vi "Waveform 64-128 channels LP pt by pt.vi"(6 "order":i32=2, 8 "fl":dbl, 10 "fs":dbl, 11 "Array in":waveform(dbl)[](array[waveform])) -> (3 "Array out":waveform(dbl)[](array[waveform]))   [LabVIEW 2016]
uses:
  <vilib>/Analysis/3filter.llb/Filter Passband Type.ctl
  <vilib>/ptbypt/NI_PtbyPt.lvlib
  <vilib>/Analysis/NI_AALBase.lvlib
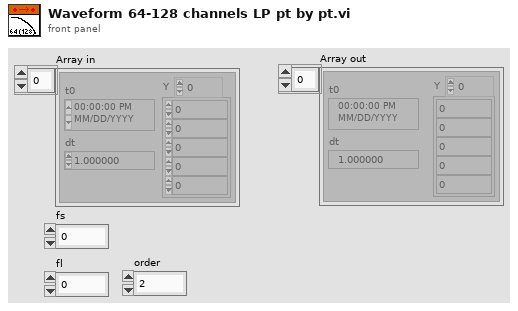
[diagram p1: front panel]
types:
  T1 = typedef "NI_AALBase.lvlib/Filter Passband Type.ctl" = enum32{"Lowpass", "Highpass", "Bandpass", "Bandstop"}
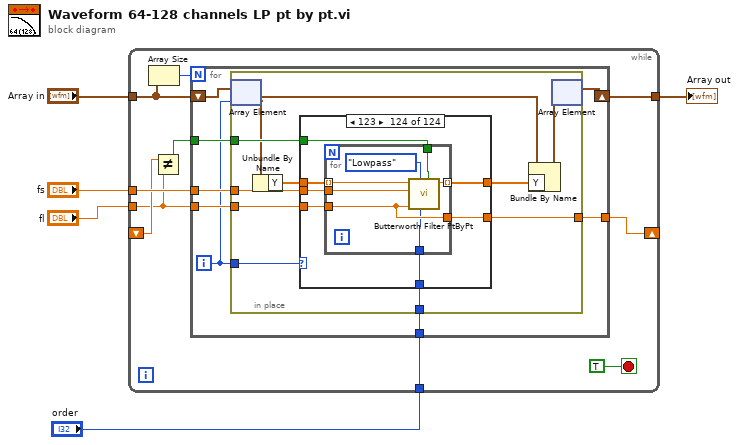
[diagram p0: block diagram]
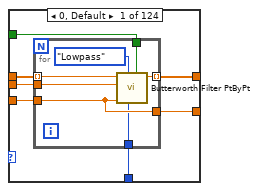
[diagram p2: hidden frame]
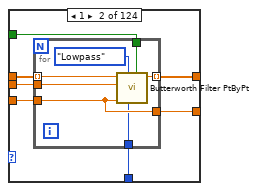
[diagram p3: hidden frame]
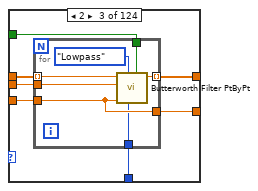
[diagram p4: hidden frame]
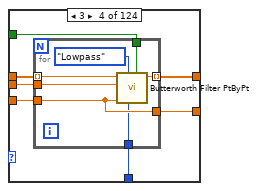
[diagram p5: hidden frame]
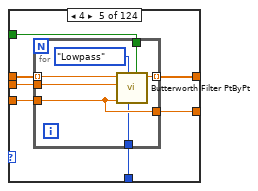
[diagram p6: hidden frame]
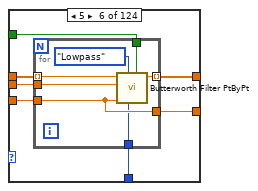
[diagram p7: hidden frame]
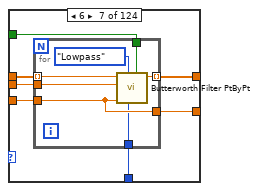
[diagram p8: hidden frame]
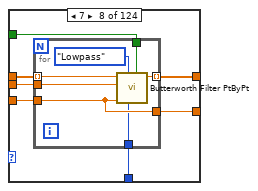
[diagram p9: hidden frame]
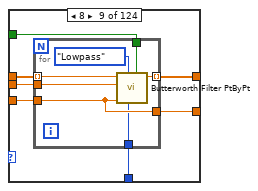
[diagram p10: hidden frame]
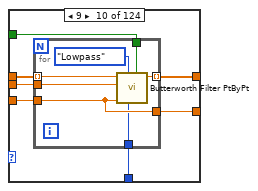
[diagram p11: hidden frame]
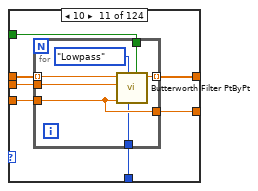
[diagram p12: hidden frame]
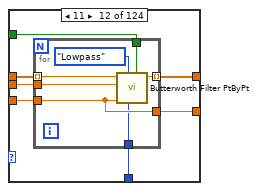
[diagram p13: hidden frame]
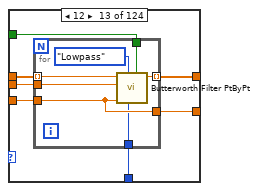
[diagram p14: hidden frame]
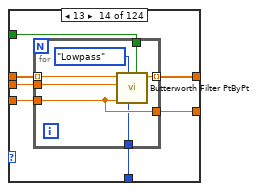
[diagram p15: hidden frame]
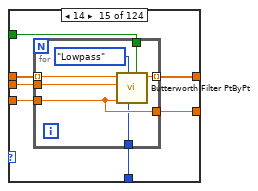
[diagram p16: hidden frame]
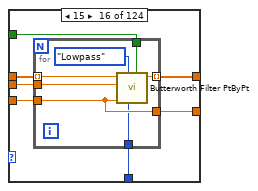
[diagram p17: hidden frame]
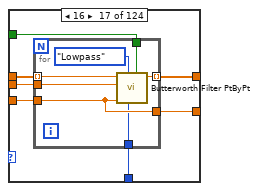
[diagram p18: hidden frame]
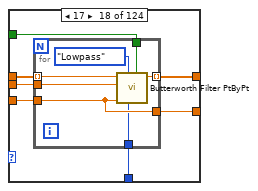
[diagram p19: hidden frame]
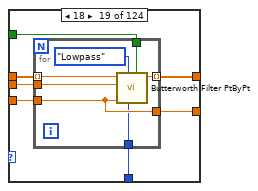
[diagram p20: hidden frame]
diagram:
  n1 = while {
    tunnel: "Array in" -> [w6]
    tunnel: [w15] -> w4
    tunnel: "fs" -> [w12]
    tunnel: "fl" -> [w9]
    shift-right: [w13] -> _
    shift-left: _ -> [w11]
    tunnel: "order" -> [w10]
    stop <- TRUE stop-if-true
    n2 = Array Size(array=w6) -> (size(s)=w7:i32)
    n3 = Not Equal?(x=w11, y=w9) -> (x != y?=w8:bool)
    n4 = for {
      N: w7 -> [_]
      tunnel: w12 -> [w23]
      tunnel: w9 -> [w22]
      tunnel: [w21] -> w13
      tunnel: w8 -> [w20]
      tunnel: w10 -> [w19]
      shift-right: [w16] -> w15
      shift-left: w6 -> [w18]
      i -> [w17]
      n5 = in-place {
        in-place-border: w23 -> [w33]
        in-place-border: w22 -> [w32]
        in-place-border: [w31] -> w21
        in-place-border: w20 -> [w30]
        in-place-border: w19 -> [w29]
        in-place-border: w17 -> [w26]
        n6 = in-place-array #1(w18, w17) -> (w25:waveform(dbl))
        n7 = Unbundle By Name(w25) -> ("Y"=w27:dbl[])
        n8 = case shown="123" w26 {
          tunnel: w33 -> [w40 w54 w68 w82 w96 w110 w124 w138 w152 w166 w180 w194 w208 w222 w236 w250 w264 w278 w292 w306 w320 w334 w348 w362 w376 w390 w404 w418 w432 w446 w460 w474 w488 w502 w516 w530 w544 w558 w572 w586 w600 w614 w628 w642 w656 w670 w684 w698 w712 w726 w740 w754 w768 w782 w796 w810 w824 w838 w852 w866 w880 w894 w908 w922 w936 w950 w964 w978 w992 w1006 w1020 w1034 w1048 w1062 w1076 w1090 w1104 w1118 w1132 w1146 w1160 w1174 w1188 w1202 w1216 w1230 w1244 w1258 w1272 w1286 w1300 w1314 w1328 w1342 w1356 w1370 w1384 w1398 w1412 w1426 w1440 w1454 w1468 w1482 w1496 w1510 w1524 w1538 w1552 w1566 w1580 w1594 w1608 w1622 w1636 w1650 w1664 w1678 w1692 w1706 w1720 w1734 w1748 w1762]
          tunnel: w32 -> [w39 w53 w67 w81 w95 w109 w123 w137 w151 w165 w179 w193 w207 w221 w235 w249 w263 w277 w291 w305 w319 w333 w347 w361 w375 w389 w403 w417 w431 w445 w459 w473 w487 w501 w515 w529 w543 w557 w571 w585 w599 w613 w627 w641 w655 w669 w683 w697 w711 w725 w739 w753 w767 w781 w795 w809 w823 w837 w851 w865 w879 w893 w907 w921 w935 w949 w963 w977 w991 w1005 w1019 w1033 w1047 w1061 w1075 w1089 w1103 w1117 w1131 w1145 w1159 w1173 w1187 w1201 w1215 w1229 w1243 w1257 w1271 w1285 w1299 w1313 w1327 w1341 w1355 w1369 w1383 w1397 w1411 w1425 w1439 w1453 w1467 w1481 w1495 w1509 w1523 w1537 w1551 w1565 w1579 w1593 w1607 w1621 w1635 w1649 w1663 w1677 w1691 w1705 w1719 w1733 w1747 w1761]
          tunnel: [w38 w52 w66 w80 w94 w108 w122 w136 w150 w164 w178 w192 w206 w220 w234 w248 w262 w276 w290 w304 w318 w332 w346 w360 w374 w388 w402 w416 w430 w444 w458 w472 w486 w500 w514 w528 w542 w556 w570 w584 w598 w612 w626 w640 w654 w668 w682 w696 w710 w724 w738 w752 w766 w780 w794 w808 w822 w836 w850 w864 w878 w892 w906 w920 w934 w948 w962 w976 w990 w1004 w1018 w1032 w1046 w1060 w1074 w1088 w1102 w1116 w1130 w1144 w1158 w1172 w1186 w1200 w1214 w1228 w1242 w1256 w1270 w1284 w1298 w1312 w1326 w1340 w1354 w1368 w1382 w1396 w1410 w1424 w1438 w1452 w1466 w1480 w1494 w1508 w1522 w1536 w1550 w1564 w1578 w1592 w1606 w1620 w1634 w1648 w1662 w1676 w1690 w1704 w1718 w1732 w1746 w1760] -> w31
          tunnel: w30 -> [w37 w51 w65 w79 w93 w107 w121 w135 w149 w163 w177 w191 w205 w219 w233 w247 w261 w275 w289 w303 w317 w331 w345 w359 w373 w387 w401 w415 w429 w443 w457 w471 w485 w499 w513 w527 w541 w555 w569 w583 w597 w611 w625 w639 w653 w667 w681 w695 w709 w723 w737 w751 w765 w779 w793 w807 w821 w835 w849 w863 w877 w891 w905 w919 w933 w947 w961 w975 w989 w1003 w1017 w1031 w1045 w1059 w1073 w1087 w1101 w1115 w1129 w1143 w1157 w1171 w1185 w1199 w1213 w1227 w1241 w1255 w1269 w1283 w1297 w1311 w1325 w1339 w1353 w1367 w1381 w1395 w1409 w1423 w1437 w1451 w1465 w1479 w1493 w1507 w1521 w1535 w1549 w1563 w1577 w1591 w1605 w1619 w1633 w1647 w1661 w1675 w1689 w1703 w1717 w1731 w1745 w1759]
          tunnel: w29 -> [w36 w50 w64 w78 w92 w106 w120 w134 w148 w162 w176 w190 w204 w218 w232 w246 w260 w274 w288 w302 w316 w330 w344 w358 w372 w386 w400 w414 w428 w442 w456 w470 w484 w498 w512 w526 w540 w554 w568 w582 w596 w610 w624 w638 w652 w666 w680 w694 w708 w722 w736 w750 w764 w778 w792 w806 w820 w834 w848 w862 w876 w890 w904 w918 w932 w946 w960 w974 w988 w1002 w1016 w1030 w1044 w1058 w1072 w1086 w1100 w1114 w1128 w1142 w1156 w1170 w1184 w1198 w1212 w1226 w1240 w1254 w1268 w1282 w1296 w1310 w1324 w1338 w1352 w1366 w1380 w1394 w1408 w1422 w1436 w1450 w1464 w1478 w1492 w1506 w1520 w1534 w1548 w1562 w1576 w1590 w1604 w1618 w1632 w1646 w1660 w1674 w1688 w1702 w1716 w1730 w1744 w1758]
          tunnel: [w35 w49 w63 w77 w91 w105 w119 w133 w147 w161 w175 w189 w203 w217 w231 w245 w259 w273 w287 w301 w315 w329 w343 w357 w371 w385 w399 w413 w427 w441 w455 w469 w483 w497 w511 w525 w539 w553 w567 w581 w595 w609 w623 w637 w651 w665 w679 w693 w707 w721 w735 w749 w763 w777 w791 w805 w819 w833 w847 w861 w875 w889 w903 w917 w931 w945 w959 w973 w987 w1001 w1015 w1029 w1043 w1057 w1071 w1085 w1099 w1113 w1127 w1141 w1155 w1169 w1183 w1197 w1211 w1225 w1239 w1253 w1267 w1281 w1295 w1309 w1323 w1337 w1351 w1365 w1379 w1393 w1407 w1421 w1435 w1449 w1463 w1477 w1491 w1505 w1519 w1533 w1547 w1561 w1575 w1589 w1603 w1617 w1631 w1645 w1659 w1673 w1687 w1701 w1715 w1729 w1743 w1757] -> w28
          tunnel: w27 -> [w34 w48 w62 w76 w90 w104 w118 w132 w146 w160 w174 w188 w202 w216 w230 w244 w258 w272 w286 w300 w314 w328 w342 w356 w370 w384 w398 w412 w426 w440 w454 w468 w482 w496 w510 w524 w538 w552 w566 w580 w594 w608 w622 w636 w650 w664 w678 w692 w706 w720 w734 w748 w762 w776 w790 w804 w818 w832 w846 w860 w874 w888 w902 w916 w930 w944 w958 w972 w986 w1000 w1014 w1028 w1042 w1056 w1070 w1084 w1098 w1112 w1126 w1140 w1154 w1168 w1182 w1196 w1210 w1224 w1238 w1252 w1266 w1280 w1294 w1308 w1322 w1336 w1350 w1364 w1378 w1392 w1406 w1420 w1434 w1448 w1462 w1476 w1490 w1504 w1518 w1532 w1546 w1560 w1574 w1588 w1602 w1616 w1630 w1644 w1658 w1672 w1686 w1700 w1714 w1728 w1742 w1756]
          frame 0, Default {
            n9 = for {
              tunnel: w34 -> [w47] mode=indexing
              tunnel: w39 -> [w44]
              tunnel: w40 -> [w46]
              tunnel: [w45] -> w35 mode=indexing
              tunnel: [w44] -> w38
              tunnel: w37 -> [w42]
              tunnel: w36 -> [w41]
              n10 = call <vilib>:"Butterworth Filter PtByPt.vi"("initialize"=w42, "order"=w41, "filter type"=Filter_Passband_Type."Lowpass", "low cutoff freq: fl"=w44, "sampling freq: fs"=w46, "x"=w47) -> ("Filtered x"=w45:dbl)  [unwired: 3 in, 1 out]
            }
          }
          frame 1 {
            n11 = for {
              tunnel: w48 -> [w61] mode=indexing
              tunnel: w53 -> [w58]
              tunnel: w54 -> [w60]
              tunnel: [w59] -> w49 mode=indexing
              tunnel: [w58] -> w52
              tunnel: w51 -> [w56]
              tunnel: w50 -> [w55]
              n12 = call <vilib>:"Butterworth Filter PtByPt.vi"("initialize"=w56, "order"=w55, "filter type"=Filter_Passband_Type."Lowpass", "low cutoff freq: fl"=w58, "sampling freq: fs"=w60, "x"=w61) -> ("Filtered x"=w59:dbl)  [unwired: 3 in, 1 out]
            }
          }
          frame 2 {
            n13 = for {
              tunnel: w62 -> [w75] mode=indexing
              tunnel: w67 -> [w72]
              tunnel: w68 -> [w74]
              tunnel: [w73] -> w63 mode=indexing
              tunnel: [w72] -> w66
              tunnel: w65 -> [w70]
              tunnel: w64 -> [w69]
              n14 = call <vilib>:"Butterworth Filter PtByPt.vi"("initialize"=w70, "order"=w69, "filter type"=Filter_Passband_Type."Lowpass", "low cutoff freq: fl"=w72, "sampling freq: fs"=w74, "x"=w75) -> ("Filtered x"=w73:dbl)  [unwired: 3 in, 1 out]
            }
          }
          frame 3 {
            n15 = for {
              tunnel: w76 -> [w89] mode=indexing
              tunnel: w81 -> [w86]
              tunnel: w82 -> [w88]
              tunnel: [w87] -> w77 mode=indexing
              tunnel: [w86] -> w80
              tunnel: w79 -> [w84]
              tunnel: w78 -> [w83]
              n16 = call <vilib>:"Butterworth Filter PtByPt.vi"("initialize"=w84, "order"=w83, "filter type"=Filter_Passband_Type."Lowpass", "low cutoff freq: fl"=w86, "sampling freq: fs"=w88, "x"=w89) -> ("Filtered x"=w87:dbl)  [unwired: 3 in, 1 out]
            }
          }
          frame 4 {
            n17 = for {
              tunnel: w90 -> [w103] mode=indexing
              tunnel: w95 -> [w100]
              tunnel: w96 -> [w102]
              tunnel: [w101] -> w91 mode=indexing
              tunnel: [w100] -> w94
              tunnel: w93 -> [w98]
              tunnel: w92 -> [w97]
              n18 = call <vilib>:"Butterworth Filter PtByPt.vi"("initialize"=w98, "order"=w97, "filter type"=Filter_Passband_Type."Lowpass", "low cutoff freq: fl"=w100, "sampling freq: fs"=w102, "x"=w103) -> ("Filtered x"=w101:dbl)  [unwired: 3 in, 1 out]
            }
          }
          frame 5 {
            n19 = for {
              tunnel: w104 -> [w117] mode=indexing
              tunnel: w109 -> [w114]
              tunnel: w110 -> [w116]
              tunnel: [w115] -> w105 mode=indexing
              tunnel: [w114] -> w108
              tunnel: w107 -> [w112]
              tunnel: w106 -> [w111]
              n20 = call <vilib>:"Butterworth Filter PtByPt.vi"("initialize"=w112, "order"=w111, "filter type"=Filter_Passband_Type."Lowpass", "low cutoff freq: fl"=w114, "sampling freq: fs"=w116, "x"=w117) -> ("Filtered x"=w115:dbl)  [unwired: 3 in, 1 out]
            }
          }
          frame 6 {
            n21 = for {
              tunnel: w118 -> [w131] mode=indexing
              tunnel: w123 -> [w128]
              tunnel: w124 -> [w130]
              tunnel: [w129] -> w119 mode=indexing
              tunnel: [w128] -> w122
              tunnel: w121 -> [w126]
              tunnel: w120 -> [w125]
              n22 = call <vilib>:"Butterworth Filter PtByPt.vi"("initialize"=w126, "order"=w125, "filter type"=Filter_Passband_Type."Lowpass", "low cutoff freq: fl"=w128, "sampling freq: fs"=w130, "x"=w131) -> ("Filtered x"=w129:dbl)  [unwired: 3 in, 1 out]
            }
          }
          frame 7 {
            n23 = for {
              tunnel: w132 -> [w145] mode=indexing
              tunnel: w137 -> [w142]
              tunnel: w138 -> [w144]
              tunnel: [w143] -> w133 mode=indexing
              tunnel: [w142] -> w136
              tunnel: w135 -> [w140]
              tunnel: w134 -> [w139]
              n24 = call <vilib>:"Butterworth Filter PtByPt.vi"("initialize"=w140, "order"=w139, "filter type"=Filter_Passband_Type."Lowpass", "low cutoff freq: fl"=w142, "sampling freq: fs"=w144, "x"=w145) -> ("Filtered x"=w143:dbl)  [unwired: 3 in, 1 out]
            }
          }
          frame 8 {
            n25 = for {
              tunnel: w146 -> [w159] mode=indexing
              tunnel: w151 -> [w156]
              tunnel: w152 -> [w158]
              tunnel: [w157] -> w147 mode=indexing
              tunnel: [w156] -> w150
              tunnel: w149 -> [w154]
              tunnel: w148 -> [w153]
              n26 = call <vilib>:"Butterworth Filter PtByPt.vi"("initialize"=w154, "order"=w153, "filter type"=Filter_Passband_Type."Lowpass", "low cutoff freq: fl"=w156, "sampling freq: fs"=w158, "x"=w159) -> ("Filtered x"=w157:dbl)  [unwired: 3 in, 1 out]
            }
          }
          frame 9 {
            n27 = for {
              tunnel: w160 -> [w173] mode=indexing
              tunnel: w165 -> [w170]
              tunnel: w166 -> [w172]
              tunnel: [w171] -> w161 mode=indexing
              tunnel: [w170] -> w164
              tunnel: w163 -> [w168]
              tunnel: w162 -> [w167]
              n28 = call <vilib>:"Butterworth Filter PtByPt.vi"("initialize"=w168, "order"=w167, "filter type"=Filter_Passband_Type."Lowpass", "low cutoff freq: fl"=w170, "sampling freq: fs"=w172, "x"=w173) -> ("Filtered x"=w171:dbl)  [unwired: 3 in, 1 out]
            }
          }
          frame 10 {
            n29 = for {
              tunnel: w174 -> [w187] mode=indexing
              tunnel: w179 -> [w184]
              tunnel: w180 -> [w186]
              tunnel: [w185] -> w175 mode=indexing
              tunnel: [w184] -> w178
              tunnel: w177 -> [w182]
              tunnel: w176 -> [w181]
              n30 = call <vilib>:"Butterworth Filter PtByPt.vi"("initialize"=w182, "order"=w181, "filter type"=Filter_Passband_Type."Lowpass", "low cutoff freq: fl"=w184, "sampling freq: fs"=w186, "x"=w187) -> ("Filtered x"=w185:dbl)  [unwired: 3 in, 1 out]
            }
          }
          frame 11 {
            n31 = for {
              tunnel: w188 -> [w201] mode=indexing
              tunnel: w193 -> [w198]
              tunnel: w194 -> [w200]
              tunnel: [w199] -> w189 mode=indexing
              tunnel: [w198] -> w192
              tunnel: w191 -> [w196]
              tunnel: w190 -> [w195]
              n32 = call <vilib>:"Butterworth Filter PtByPt.vi"("initialize"=w196, "order"=w195, "filter type"=Filter_Passband_Type."Lowpass", "low cutoff freq: fl"=w198, "sampling freq: fs"=w200, "x"=w201) -> ("Filtered x"=w199:dbl)  [unwired: 3 in, 1 out]
            }
          }
          frame 12 {
            n33 = for {
              tunnel: w202 -> [w215] mode=indexing
              tunnel: w207 -> [w212]
              tunnel: w208 -> [w214]
              tunnel: [w213] -> w203 mode=indexing
              tunnel: [w212] -> w206
              tunnel: w205 -> [w210]
              tunnel: w204 -> [w209]
              n34 = call <vilib>:"Butterworth Filter PtByPt.vi"("initialize"=w210, "order"=w209, "filter type"=Filter_Passband_Type."Lowpass", "low cutoff freq: fl"=w212, "sampling freq: fs"=w214, "x"=w215) -> ("Filtered x"=w213:dbl)  [unwired: 3 in, 1 out]
            }
          }
          frame 13 {
            n35 = for {
              tunnel: w216 -> [w229] mode=indexing
              tunnel: w221 -> [w226]
              tunnel: w222 -> [w228]
              tunnel: [w227] -> w217 mode=indexing
              tunnel: [w226] -> w220
              tunnel: w219 -> [w224]
              tunnel: w218 -> [w223]
              n36 = call <vilib>:"Butterworth Filter PtByPt.vi"("initialize"=w224, "order"=w223, "filter type"=Filter_Passband_Type."Lowpass", "low cutoff freq: fl"=w226, "sampling freq: fs"=w228, "x"=w229) -> ("Filtered x"=w227:dbl)  [unwired: 3 in, 1 out]
            }
          }
          frame 14 {
            n37 = for {
              tunnel: w230 -> [w243] mode=indexing
              tunnel: w235 -> [w240]
              tunnel: w236 -> [w242]
              tunnel: [w241] -> w231 mode=indexing
              tunnel: [w240] -> w234
              tunnel: w233 -> [w238]
              tunnel: w232 -> [w237]
              n38 = call <vilib>:"Butterworth Filter PtByPt.vi"("initialize"=w238, "order"=w237, "filter type"=Filter_Passband_Type."Lowpass", "low cutoff freq: fl"=w240, "sampling freq: fs"=w242, "x"=w243) -> ("Filtered x"=w241:dbl)  [unwired: 3 in, 1 out]
            }
          }
          frame 15 {
            n39 = for {
              tunnel: w244 -> [w257] mode=indexing
              tunnel: w249 -> [w254]
              tunnel: w250 -> [w256]
              tunnel: [w255] -> w245 mode=indexing
              tunnel: [w254] -> w248
              tunnel: w247 -> [w252]
              tunnel: w246 -> [w251]
              n40 = call <vilib>:"Butterworth Filter PtByPt.vi"("initialize"=w252, "order"=w251, "filter type"=Filter_Passband_Type."Lowpass", "low cutoff freq: fl"=w254, "sampling freq: fs"=w256, "x"=w257) -> ("Filtered x"=w255:dbl)  [unwired: 3 in, 1 out]
            }
          }
          frame 16 {
            n41 = for {
              tunnel: w258 -> [w271] mode=indexing
              tunnel: w263 -> [w268]
              tunnel: w264 -> [w270]
              tunnel: [w269] -> w259 mode=indexing
              tunnel: [w268] -> w262
              tunnel: w261 -> [w266]
              tunnel: w260 -> [w265]
              n42 = call <vilib>:"Butterworth Filter PtByPt.vi"("initialize"=w266, "order"=w265, "filter type"=Filter_Passband_Type."Lowpass", "low cutoff freq: fl"=w268, "sampling freq: fs"=w270, "x"=w271) -> ("Filtered x"=w269:dbl)  [unwired: 3 in, 1 out]
            }
          }
          frame 17 {
            n43 = for {
              tunnel: w272 -> [w285] mode=indexing
              tunnel: w277 -> [w282]
              tunnel: w278 -> [w284]
              tunnel: [w283] -> w273 mode=indexing
              tunnel: [w282] -> w276
              tunnel: w275 -> [w280]
              tunnel: w274 -> [w279]
              n44 = call <vilib>:"Butterworth Filter PtByPt.vi"("initialize"=w280, "order"=w279, "filter type"=Filter_Passband_Type."Lowpass", "low cutoff freq: fl"=w282, "sampling freq: fs"=w284, "x"=w285) -> ("Filtered x"=w283:dbl)  [unwired: 3 in, 1 out]
            }
          }
          frame 18 {
            n45 = for {
              tunnel: w286 -> [w299] mode=indexing
              tunnel: w291 -> [w296]
              tunnel: w292 -> [w298]
              tunnel: [w297] -> w287 mode=indexing
              tunnel: [w296] -> w290
              tunnel: w289 -> [w294]
              tunnel: w288 -> [w293]
              n46 = call <vilib>:"Butterworth Filter PtByPt.vi"("initialize"=w294, "order"=w293, "filter type"=Filter_Passband_Type."Lowpass", "low cutoff freq: fl"=w296, "sampling freq: fs"=w298, "x"=w299) -> ("Filtered x"=w297:dbl)  [unwired: 3 in, 1 out]
            }
          }
          frame 19 {
            n47 = for {
              tunnel: w300 -> [w313] mode=indexing
              tunnel: w305 -> [w310]
              tunnel: w306 -> [w312]
              tunnel: [w311] -> w301 mode=indexing
              tunnel: [w310] -> w304
              tunnel: w303 -> [w308]
              tunnel: w302 -> [w307]
              n48 = call <vilib>:"Butterworth Filter PtByPt.vi"("initialize"=w308, "order"=w307, "filter type"=Filter_Passband_Type."Lowpass", "low cutoff freq: fl"=w310, "sampling freq: fs"=w312, "x"=w313) -> ("Filtered x"=w311:dbl)  [unwired: 3 in, 1 out]
            }
          }
          frame 20 {
            n49 = for {
              tunnel: w314 -> [w327] mode=indexing
              tunnel: w319 -> [w324]
              tunnel: w320 -> [w326]
              tunnel: [w325] -> w315 mode=indexing
              tunnel: [w324] -> w318
              tunnel: w317 -> [w322]
              tunnel: w316 -> [w321]
              n50 = call <vilib>:"Butterworth Filter PtByPt.vi"("initialize"=w322, "order"=w321, "filter type"=Filter_Passband_Type."Lowpass", "low cutoff freq: fl"=w324, "sampling freq: fs"=w326, "x"=w327) -> ("Filtered x"=w325:dbl)  [unwired: 3 in, 1 out]
            }
          }
          frame 21 {
            n51 = for {
              tunnel: w328 -> [w341] mode=indexing
              tunnel: w333 -> [w338]
              tunnel: w334 -> [w340]
              tunnel: [w339] -> w329 mode=indexing
              tunnel: [w338] -> w332
              tunnel: w331 -> [w336]
              tunnel: w330 -> [w335]
              n52 = call <vilib>:"Butterworth Filter PtByPt.vi"("initialize"=w336, "order"=w335, "filter type"=Filter_Passband_Type."Lowpass", "low cutoff freq: fl"=w338, "sampling freq: fs"=w340, "x"=w341) -> ("Filtered x"=w339:dbl)  [unwired: 3 in, 1 out]
            }
          }
          frame 22 {
            n53 = for {
              tunnel: w342 -> [w355] mode=indexing
              tunnel: w347 -> [w352]
              tunnel: w348 -> [w354]
              tunnel: [w353] -> w343 mode=indexing
              tunnel: [w352] -> w346
              tunnel: w345 -> [w350]
              tunnel: w344 -> [w349]
              n54 = call <vilib>:"Butterworth Filter PtByPt.vi"("initialize"=w350, "order"=w349, "filter type"=Filter_Passband_Type."Lowpass", "low cutoff freq: fl"=w352, "sampling freq: fs"=w354, "x"=w355) -> ("Filtered x"=w353:dbl)  [unwired: 3 in, 1 out]
            }
          }
          frame 23 {
            n55 = for {
              tunnel: w356 -> [w369] mode=indexing
              tunnel: w361 -> [w366]
              tunnel: w362 -> [w368]
              tunnel: [w367] -> w357 mode=indexing
              tunnel: [w366] -> w360
              tunnel: w359 -> [w364]
              tunnel: w358 -> [w363]
              n56 = call <vilib>:"Butterworth Filter PtByPt.vi"("initialize"=w364, "order"=w363, "filter type"=Filter_Passband_Type."Lowpass", "low cutoff freq: fl"=w366, "sampling freq: fs"=w368, "x"=w369) -> ("Filtered x"=w367:dbl)  [unwired: 3 in, 1 out]
            }
          }
          frame 24 {
            n57 = for {
              tunnel: w370 -> [w383] mode=indexing
              tunnel: w375 -> [w380]
              tunnel: w376 -> [w382]
              tunnel: [w381] -> w371 mode=indexing
              tunnel: [w380] -> w374
              tunnel: w373 -> [w378]
              tunnel: w372 -> [w377]
              n58 = call <vilib>:"Butterworth Filter PtByPt.vi"("initialize"=w378, "order"=w377, "filter type"=Filter_Passband_Type."Lowpass", "low cutoff freq: fl"=w380, "sampling freq: fs"=w382, "x"=w383) -> ("Filtered x"=w381:dbl)  [unwired: 3 in, 1 out]
            }
          }
          frame 25 {
            n59 = for {
              tunnel: w384 -> [w397] mode=indexing
              tunnel: w389 -> [w394]
              tunnel: w390 -> [w396]
              tunnel: [w395] -> w385 mode=indexing
              tunnel: [w394] -> w388
              tunnel: w387 -> [w392]
              tunnel: w386 -> [w391]
              n60 = call <vilib>:"Butterworth Filter PtByPt.vi"("initialize"=w392, "order"=w391, "filter type"=Filter_Passband_Type."Lowpass", "low cutoff freq: fl"=w394, "sampling freq: fs"=w396, "x"=w397) -> ("Filtered x"=w395:dbl)  [unwired: 3 in, 1 out]
            }
          }
          frame 26 {
            n61 = for {
              tunnel: w398 -> [w411] mode=indexing
              tunnel: w403 -> [w408]
              tunnel: w404 -> [w410]
              tunnel: [w409] -> w399 mode=indexing
              tunnel: [w408] -> w402
              tunnel: w401 -> [w406]
              tunnel: w400 -> [w405]
              n62 = call <vilib>:"Butterworth Filter PtByPt.vi"("initialize"=w406, "order"=w405, "filter type"=Filter_Passband_Type."Lowpass", "low cutoff freq: fl"=w408, "sampling freq: fs"=w410, "x"=w411) -> ("Filtered x"=w409:dbl)  [unwired: 3 in, 1 out]
            }
          }
          frame 27 {
            n63 = for {
              tunnel: w412 -> [w425] mode=indexing
              tunnel: w417 -> [w422]
              tunnel: w418 -> [w424]
              tunnel: [w423] -> w413 mode=indexing
              tunnel: [w422] -> w416
              tunnel: w415 -> [w420]
              tunnel: w414 -> [w419]
              n64 = call <vilib>:"Butterworth Filter PtByPt.vi"("initialize"=w420, "order"=w419, "filter type"=Filter_Passband_Type."Lowpass", "low cutoff freq: fl"=w422, "sampling freq: fs"=w424, "x"=w425) -> ("Filtered x"=w423:dbl)  [unwired: 3 in, 1 out]
            }
          }
          frame 28 {
            n65 = for {
              tunnel: w426 -> [w439] mode=indexing
              tunnel: w431 -> [w436]
              tunnel: w432 -> [w438]
              tunnel: [w437] -> w427 mode=indexing
              tunnel: [w436] -> w430
              tunnel: w429 -> [w434]
              tunnel: w428 -> [w433]
              n66 = call <vilib>:"Butterworth Filter PtByPt.vi"("initialize"=w434, "order"=w433, "filter type"=Filter_Passband_Type."Lowpass", "low cutoff freq: fl"=w436, "sampling freq: fs"=w438, "x"=w439) -> ("Filtered x"=w437:dbl)  [unwired: 3 in, 1 out]
            }
          }
          frame 29 {
            n67 = for {
              tunnel: w440 -> [w453] mode=indexing
              tunnel: w445 -> [w450]
              tunnel: w446 -> [w452]
              tunnel: [w451] -> w441 mode=indexing
              tunnel: [w450] -> w444
              tunnel: w443 -> [w448]
              tunnel: w442 -> [w447]
              n68 = call <vilib>:"Butterworth Filter PtByPt.vi"("initialize"=w448, "order"=w447, "filter type"=Filter_Passband_Type."Lowpass", "low cutoff freq: fl"=w450, "sampling freq: fs"=w452, "x"=w453) -> ("Filtered x"=w451:dbl)  [unwired: 3 in, 1 out]
            }
          }
          frame 30 {
            n69 = for {
              tunnel: w454 -> [w467] mode=indexing
              tunnel: w459 -> [w464]
              tunnel: w460 -> [w466]
              tunnel: [w465] -> w455 mode=indexing
              tunnel: [w464] -> w458
              tunnel: w457 -> [w462]
              tunnel: w456 -> [w461]
              n70 = call <vilib>:"Butterworth Filter PtByPt.vi"("initialize"=w462, "order"=w461, "filter type"=Filter_Passband_Type."Lowpass", "low cutoff freq: fl"=w464, "sampling freq: fs"=w466, "x"=w467) -> ("Filtered x"=w465:dbl)  [unwired: 3 in, 1 out]
            }
          }
          frame 31 {
            n71 = for {
              tunnel: w468 -> [w481] mode=indexing
              tunnel: w473 -> [w478]
              tunnel: w474 -> [w480]
              tunnel: [w479] -> w469 mode=indexing
              tunnel: [w478] -> w472
              tunnel: w471 -> [w476]
              tunnel: w470 -> [w475]
              n72 = call <vilib>:"Butterworth Filter PtByPt.vi"("initialize"=w476, "order"=w475, "filter type"=Filter_Passband_Type."Lowpass", "low cutoff freq: fl"=w478, "sampling freq: fs"=w480, "x"=w481) -> ("Filtered x"=w479:dbl)  [unwired: 3 in, 1 out]
            }
          }
          frame 32 {
            n73 = for {
              tunnel: w482 -> [w495] mode=indexing
              tunnel: w487 -> [w492]
              tunnel: w488 -> [w494]
              tunnel: [w493] -> w483 mode=indexing
              tunnel: [w492] -> w486
              tunnel: w485 -> [w490]
              tunnel: w484 -> [w489]
              n74 = call <vilib>:"Butterworth Filter PtByPt.vi"("initialize"=w490, "order"=w489, "filter type"=Filter_Passband_Type."Lowpass", "low cutoff freq: fl"=w492, "sampling freq: fs"=w494, "x"=w495) -> ("Filtered x"=w493:dbl)  [unwired: 3 in, 1 out]
            }
          }
          frame 33 {
            n75 = for {
              tunnel: w496 -> [w509] mode=indexing
              tunnel: w501 -> [w506]
              tunnel: w502 -> [w508]
              tunnel: [w507] -> w497 mode=indexing
              tunnel: [w506] -> w500
              tunnel: w499 -> [w504]
              tunnel: w498 -> [w503]
              n76 = call <vilib>:"Butterworth Filter PtByPt.vi"("initialize"=w504, "order"=w503, "filter type"=Filter_Passband_Type."Lowpass", "low cutoff freq: fl"=w506, "sampling freq: fs"=w508, "x"=w509) -> ("Filtered x"=w507:dbl)  [unwired: 3 in, 1 out]
            }
          }
          frame 34 {
            n77 = for {
              tunnel: w510 -> [w523] mode=indexing
              tunnel: w515 -> [w520]
              tunnel: w516 -> [w522]
              tunnel: [w521] -> w511 mode=indexing
              tunnel: [w520] -> w514
              tunnel: w513 -> [w518]
              tunnel: w512 -> [w517]
              n78 = call <vilib>:"Butterworth Filter PtByPt.vi"("initialize"=w518, "order"=w517, "filter type"=Filter_Passband_Type."Lowpass", "low cutoff freq: fl"=w520, "sampling freq: fs"=w522, "x"=w523) -> ("Filtered x"=w521:dbl)  [unwired: 3 in, 1 out]
            }
          }
          frame 35 {
            n79 = for {
              tunnel: w524 -> [w537] mode=indexing
              tunnel: w529 -> [w534]
              tunnel: w530 -> [w536]
              tunnel: [w535] -> w525 mode=indexing
              tunnel: [w534] -> w528
              tunnel: w527 -> [w532]
              tunnel: w526 -> [w531]
              n80 = call <vilib>:"Butterworth Filter PtByPt.vi"("initialize"=w532, "order"=w531, "filter type"=Filter_Passband_Type."Lowpass", "low cutoff freq: fl"=w534, "sampling freq: fs"=w536, "x"=w537) -> ("Filtered x"=w535:dbl)  [unwired: 3 in, 1 out]
            }
          }
          frame 36 {
            n81 = for {
              tunnel: w538 -> [w551] mode=indexing
              tunnel: w543 -> [w548]
              tunnel: w544 -> [w550]
              tunnel: [w549] -> w539 mode=indexing
              tunnel: [w548] -> w542
              tunnel: w541 -> [w546]
              tunnel: w540 -> [w545]
              n82 = call <vilib>:"Butterworth Filter PtByPt.vi"("initialize"=w546, "order"=w545, "filter type"=Filter_Passband_Type."Lowpass", "low cutoff freq: fl"=w548, "sampling freq: fs"=w550, "x"=w551) -> ("Filtered x"=w549:dbl)  [unwired: 3 in, 1 out]
            }
          }
          frame 37 {
            n83 = for {
              tunnel: w552 -> [w565] mode=indexing
              tunnel: w557 -> [w562]
              tunnel: w558 -> [w564]
              tunnel: [w563] -> w553 mode=indexing
              tunnel: [w562] -> w556
              tunnel: w555 -> [w560]
              tunnel: w554 -> [w559]
              n84 = call <vilib>:"Butterworth Filter PtByPt.vi"("initialize"=w560, "order"=w559, "filter type"=Filter_Passband_Type."Lowpass", "low cutoff freq: fl"=w562, "sampling freq: fs"=w564, "x"=w565) -> ("Filtered x"=w563:dbl)  [unwired: 3 in, 1 out]
            }
          }
          frame 38 {
            n85 = for {
              tunnel: w566 -> [w579] mode=indexing
              tunnel: w571 -> [w576]
              tunnel: w572 -> [w578]
              tunnel: [w577] -> w567 mode=indexing
              tunnel: [w576] -> w570
              tunnel: w569 -> [w574]
              tunnel: w568 -> [w573]
              n86 = call <vilib>:"Butterworth Filter PtByPt.vi"("initialize"=w574, "order"=w573, "filter type"=Filter_Passband_Type."Lowpass", "low cutoff freq: fl"=w576, "sampling freq: fs"=w578, "x"=w579) -> ("Filtered x"=w577:dbl)  [unwired: 3 in, 1 out]
            }
          }
          frame 39 {
            n87 = for {
              tunnel: w580 -> [w593] mode=indexing
              tunnel: w585 -> [w590]
              tunnel: w586 -> [w592]
              tunnel: [w591] -> w581 mode=indexing
              tunnel: [w590] -> w584
              tunnel: w583 -> [w588]
              tunnel: w582 -> [w587]
              n88 = call <vilib>:"Butterworth Filter PtByPt.vi"("initialize"=w588, "order"=w587, "filter type"=Filter_Passband_Type."Lowpass", "low cutoff freq: fl"=w590, "sampling freq: fs"=w592, "x"=w593) -> ("Filtered x"=w591:dbl)  [unwired: 3 in, 1 out]
            }
          }
          frame 40 {
            n89 = for {
              tunnel: w594 -> [w607] mode=indexing
              tunnel: w599 -> [w604]
              tunnel: w600 -> [w606]
              tunnel: [w605] -> w595 mode=indexing
              tunnel: [w604] -> w598
              tunnel: w597 -> [w602]
              tunnel: w596 -> [w601]
              n90 = call <vilib>:"Butterworth Filter PtByPt.vi"("initialize"=w602, "order"=w601, "filter type"=Filter_Passband_Type."Lowpass", "low cutoff freq: fl"=w604, "sampling freq: fs"=w606, "x"=w607) -> ("Filtered x"=w605:dbl)  [unwired: 3 in, 1 out]
            }
          }
          frame 41 {
            n91 = for {
              tunnel: w608 -> [w621] mode=indexing
              tunnel: w613 -> [w618]
              tunnel: w614 -> [w620]
              tunnel: [w619] -> w609 mode=indexing
              tunnel: [w618] -> w612
              tunnel: w611 -> [w616]
              tunnel: w610 -> [w615]
              n92 = call <vilib>:"Butterworth Filter PtByPt.vi"("initialize"=w616, "order"=w615, "filter type"=Filter_Passband_Type."Lowpass", "low cutoff freq: fl"=w618, "sampling freq: fs"=w620, "x"=w621) -> ("Filtered x"=w619:dbl)  [unwired: 3 in, 1 out]
            }
          }
          frame 42 {
            n93 = for {
              tunnel: w622 -> [w635] mode=indexing
              tunnel: w627 -> [w632]
              tunnel: w628 -> [w634]
              tunnel: [w633] -> w623 mode=indexing
              tunnel: [w632] -> w626
              tunnel: w625 -> [w630]
              tunnel: w624 -> [w629]
              n94 = call <vilib>:"Butterworth Filter PtByPt.vi"("initialize"=w630, "order"=w629, "filter type"=Filter_Passband_Type."Lowpass", "low cutoff freq: fl"=w632, "sampling freq: fs"=w634, "x"=w635) -> ("Filtered x"=w633:dbl)  [unwired: 3 in, 1 out]
            }
          }
          frame 43 {
            n95 = for {
              tunnel: w636 -> [w649] mode=indexing
              tunnel: w641 -> [w646]
              tunnel: w642 -> [w648]
              tunnel: [w647] -> w637 mode=indexing
              tunnel: [w646] -> w640
              tunnel: w639 -> [w644]
              tunnel: w638 -> [w643]
              n96 = call <vilib>:"Butterworth Filter PtByPt.vi"("initialize"=w644, "order"=w643, "filter type"=Filter_Passband_Type."Lowpass", "low cutoff freq: fl"=w646, "sampling freq: fs"=w648, "x"=w649) -> ("Filtered x"=w647:dbl)  [unwired: 3 in, 1 out]
            }
          }
          frame 44 {
            n97 = for {
              tunnel: w650 -> [w663] mode=indexing
              tunnel: w655 -> [w660]
              tunnel: w656 -> [w662]
              tunnel: [w661] -> w651 mode=indexing
              tunnel: [w660] -> w654
              tunnel: w653 -> [w658]
              tunnel: w652 -> [w657]
              n98 = call <vilib>:"Butterworth Filter PtByPt.vi"("initialize"=w658, "order"=w657, "filter type"=Filter_Passband_Type."Lowpass", "low cutoff freq: fl"=w660, "sampling freq: fs"=w662, "x"=w663) -> ("Filtered x"=w661:dbl)  [unwired: 3 in, 1 out]
            }
          }
          frame 45 {
            n99 = for {
              tunnel: w664 -> [w677] mode=indexing
              tunnel: w669 -> [w674]
              tunnel: w670 -> [w676]
              tunnel: [w675] -> w665 mode=indexing
              tunnel: [w674] -> w668
              tunnel: w667 -> [w672]
              tunnel: w666 -> [w671]
              n100 = call <vilib>:"Butterworth Filter PtByPt.vi"("initialize"=w672, "order"=w671, "filter type"=Filter_Passband_Type."Lowpass", "low cutoff freq: fl"=w674, "sampling freq: fs"=w676, "x"=w677) -> ("Filtered x"=w675:dbl)  [unwired: 3 in, 1 out]
            }
          }
          frame 46 {
            n101 = for {
              tunnel: w678 -> [w691] mode=indexing
              tunnel: w683 -> [w688]
              tunnel: w684 -> [w690]
              tunnel: [w689] -> w679 mode=indexing
              tunnel: [w688] -> w682
              tunnel: w681 -> [w686]
              tunnel: w680 -> [w685]
              n102 = call <vilib>:"Butterworth Filter PtByPt.vi"("initialize"=w686, "order"=w685, "filter type"=Filter_Passband_Type."Lowpass", "low cutoff freq: fl"=w688, "sampling freq: fs"=w690, "x"=w691) -> ("Filtered x"=w689:dbl)  [unwired: 3 in, 1 out]
            }
          }
          frame 47 {
            n103 = for {
              tunnel: w692 -> [w705] mode=indexing
              tunnel: w697 -> [w702]
              tunnel: w698 -> [w704]
              tunnel: [w703] -> w693 mode=indexing
              tunnel: [w702] -> w696
              tunnel: w695 -> [w700]
              tunnel: w694 -> [w699]
              n104 = call <vilib>:"Butterworth Filter PtByPt.vi"("initialize"=w700, "order"=w699, "filter type"=Filter_Passband_Type."Lowpass", "low cutoff freq: fl"=w702, "sampling freq: fs"=w704, "x"=w705) -> ("Filtered x"=w703:dbl)  [unwired: 3 in, 1 out]
            }
          }
          frame 48 {
            n105 = for {
              tunnel: w706 -> [w719] mode=indexing
              tunnel: w711 -> [w716]
              tunnel: w712 -> [w718]
              tunnel: [w717] -> w707 mode=indexing
              tunnel: [w716] -> w710
              tunnel: w709 -> [w714]
              tunnel: w708 -> [w713]
              n106 = call <vilib>:"Butterworth Filter PtByPt.vi"("initialize"=w714, "order"=w713, "filter type"=Filter_Passband_Type."Lowpass", "low cutoff freq: fl"=w716, "sampling freq: fs"=w718, "x"=w719) -> ("Filtered x"=w717:dbl)  [unwired: 3 in, 1 out]
            }
          }
          frame 49 {
            n107 = for {
              tunnel: w720 -> [w733] mode=indexing
              tunnel: w725 -> [w730]
              tunnel: w726 -> [w732]
              tunnel: [w731] -> w721 mode=indexing
              tunnel: [w730] -> w724
              tunnel: w723 -> [w728]
              tunnel: w722 -> [w727]
              n108 = call <vilib>:"Butterworth Filter PtByPt.vi"("initialize"=w728, "order"=w727, "filter type"=Filter_Passband_Type."Lowpass", "low cutoff freq: fl"=w730, "sampling freq: fs"=w732, "x"=w733) -> ("Filtered x"=w731:dbl)  [unwired: 3 in, 1 out]
            }
          }
          frame 50 {
            n109 = for {
              tunnel: w734 -> [w747] mode=indexing
              tunnel: w739 -> [w744]
              tunnel: w740 -> [w746]
              tunnel: [w745] -> w735 mode=indexing
              tunnel: [w744] -> w738
              tunnel: w737 -> [w742]
              tunnel: w736 -> [w741]
              n110 = call <vilib>:"Butterworth Filter PtByPt.vi"("initialize"=w742, "order"=w741, "filter type"=Filter_Passband_Type."Lowpass", "low cutoff freq: fl"=w744, "sampling freq: fs"=w746, "x"=w747) -> ("Filtered x"=w745:dbl)  [unwired: 3 in, 1 out]
            }
          }
          frame 51 {
            n111 = for {
              tunnel: w748 -> [w761] mode=indexing
              tunnel: w753 -> [w758]
              tunnel: w754 -> [w760]
              tunnel: [w759] -> w749 mode=indexing
              tunnel: [w758] -> w752
              tunnel: w751 -> [w756]
              tunnel: w750 -> [w755]
              n112 = call <vilib>:"Butterworth Filter PtByPt.vi"("initialize"=w756, "order"=w755, "filter type"=Filter_Passband_Type."Lowpass", "low cutoff freq: fl"=w758, "sampling freq: fs"=w760, "x"=w761) -> ("Filtered x"=w759:dbl)  [unwired: 3 in, 1 out]
            }
          }
          frame 52 {
            n113 = for {
              tunnel: w762 -> [w775] mode=indexing
              tunnel: w767 -> [w772]
              tunnel: w768 -> [w774]
              tunnel: [w773] -> w763 mode=indexing
              tunnel: [w772] -> w766
              tunnel: w765 -> [w770]
              tunnel: w764 -> [w769]
              n114 = call <vilib>:"Butterworth Filter PtByPt.vi"("initialize"=w770, "order"=w769, "filter type"=Filter_Passband_Type."Lowpass", "low cutoff freq: fl"=w772, "sampling freq: fs"=w774, "x"=w775) -> ("Filtered x"=w773:dbl)  [unwired: 3 in, 1 out]
            }
          }
          frame 53 {
            n115 = for {
              tunnel: w776 -> [w789] mode=indexing
              tunnel: w781 -> [w786]
              tunnel: w782 -> [w788]
              tunnel: [w787] -> w777 mode=indexing
              tunnel: [w786] -> w780
              tunnel: w779 -> [w784]
              tunnel: w778 -> [w783]
              n116 = call <vilib>:"Butterworth Filter PtByPt.vi"("initialize"=w784, "order"=w783, "filter type"=Filter_Passband_Type."Lowpass", "low cutoff freq: fl"=w786, "sampling freq: fs"=w788, "x"=w789) -> ("Filtered x"=w787:dbl)  [unwired: 3 in, 1 out]
            }
          }
          frame 54 {
            n117 = for {
              tunnel: w790 -> [w803] mode=indexing
              tunnel: w795 -> [w800]
              tunnel: w796 -> [w802]
              tunnel: [w801] -> w791 mode=indexing
              tunnel: [w800] -> w794
              tunnel: w793 -> [w798]
              tunnel: w792 -> [w797]
              n118 = call <vilib>:"Butterworth Filter PtByPt.vi"("initialize"=w798, "order"=w797, "filter type"=Filter_Passband_Type."Lowpass", "low cutoff freq: fl"=w800, "sampling freq: fs"=w802, "x"=w803) -> ("Filtered x"=w801:dbl)  [unwired: 3 in, 1 out]
            }
          }
          frame 55 {
            n119 = for {
              tunnel: w804 -> [w817] mode=indexing
              tunnel: w809 -> [w814]
              tunnel: w810 -> [w816]
              tunnel: [w815] -> w805 mode=indexing
              tunnel: [w814] -> w808
              tunnel: w807 -> [w812]
              tunnel: w806 -> [w811]
              n120 = call <vilib>:"Butterworth Filter PtByPt.vi"("initialize"=w812, "order"=w811, "filter type"=Filter_Passband_Type."Lowpass", "low cutoff freq: fl"=w814, "sampling freq: fs"=w816, "x"=w817) -> ("Filtered x"=w815:dbl)  [unwired: 3 in, 1 out]
            }
          }
          frame 56 {
            n121 = for {
              tunnel: w818 -> [w831] mode=indexing
              tunnel: w823 -> [w828]
              tunnel: w824 -> [w830]
              tunnel: [w829] -> w819 mode=indexing
              tunnel: [w828] -> w822
              tunnel: w821 -> [w826]
              tunnel: w820 -> [w825]
              n122 = call <vilib>:"Butterworth Filter PtByPt.vi"("initialize"=w826, "order"=w825, "filter type"=Filter_Passband_Type."Lowpass", "low cutoff freq: fl"=w828, "sampling freq: fs"=w830, "x"=w831) -> ("Filtered x"=w829:dbl)  [unwired: 3 in, 1 out]
            }
          }
          frame 57 {
            n123 = for {
              tunnel: w832 -> [w845] mode=indexing
              tunnel: w837 -> [w842]
              tunnel: w838 -> [w844]
              tunnel: [w843] -> w833 mode=indexing
              tunnel: [w842] -> w836
              tunnel: w835 -> [w840]
              tunnel: w834 -> [w839]
              n124 = call <vilib>:"Butterworth Filter PtByPt.vi"("initialize"=w840, "order"=w839, "filter type"=Filter_Passband_Type."Lowpass", "low cutoff freq: fl"=w842, "sampling freq: fs"=w844, "x"=w845) -> ("Filtered x"=w843:dbl)  [unwired: 3 in, 1 out]
            }
          }
          frame 58 {
            n125 = for {
              tunnel: w846 -> [w859] mode=indexing
              tunnel: w851 -> [w856]
              tunnel: w852 -> [w858]
              tunnel: [w857] -> w847 mode=indexing
              tunnel: [w856] -> w850
              tunnel: w849 -> [w854]
              tunnel: w848 -> [w853]
              n126 = call <vilib>:"Butterworth Filter PtByPt.vi"("initialize"=w854, "order"=w853, "filter type"=Filter_Passband_Type."Lowpass", "low cutoff freq: fl"=w856, "sampling freq: fs"=w858, "x"=w859) -> ("Filtered x"=w857:dbl)  [unwired: 3 in, 1 out]
            }
          }
          frame 59 {
            n127 = for {
              tunnel: w860 -> [w873] mode=indexing
              tunnel: w865 -> [w870]
              tunnel: w866 -> [w872]
              tunnel: [w871] -> w861 mode=indexing
              tunnel: [w870] -> w864
              tunnel: w863 -> [w868]
              tunnel: w862 -> [w867]
              n128 = call <vilib>:"Butterworth Filter PtByPt.vi"("initialize"=w868, "order"=w867, "filter type"=Filter_Passband_Type."Lowpass", "low cutoff freq: fl"=w870, "sampling freq: fs"=w872, "x"=w873) -> ("Filtered x"=w871:dbl)  [unwired: 3 in, 1 out]
            }
          }
          frame 60 {
            n129 = for {
              tunnel: w874 -> [w887] mode=indexing
              tunnel: w879 -> [w884]
              tunnel: w880 -> [w886]
              tunnel: [w885] -> w875 mode=indexing
              tunnel: [w884] -> w878
              tunnel: w877 -> [w882]
              tunnel: w876 -> [w881]
              n130 = call <vilib>:"Butterworth Filter PtByPt.vi"("initialize"=w882, "order"=w881, "filter type"=Filter_Passband_Type."Lowpass", "low cutoff freq: fl"=w884, "sampling freq: fs"=w886, "x"=w887) -> ("Filtered x"=w885:dbl)  [unwired: 3 in, 1 out]
            }
          }
          frame 61 {
            n131 = for {
              tunnel: w888 -> [w901] mode=indexing
              tunnel: w893 -> [w898]
              tunnel: w894 -> [w900]
              tunnel: [w899] -> w889 mode=indexing
              tunnel: [w898] -> w892
              tunnel: w891 -> [w896]
              tunnel: w890 -> [w895]
              n132 = call <vilib>:"Butterworth Filter PtByPt.vi"("initialize"=w896, "order"=w895, "filter type"=Filter_Passband_Type."Lowpass", "low cutoff freq: fl"=w898, "sampling freq: fs"=w900, "x"=w901) -> ("Filtered x"=w899:dbl)  [unwired: 3 in, 1 out]
            }
          }
          frame 62 {
            n133 = for {
              tunnel: w902 -> [w915] mode=indexing
              tunnel: w907 -> [w912]
              tunnel: w908 -> [w914]
              tunnel: [w913] -> w903 mode=indexing
              tunnel: [w912] -> w906
              tunnel: w905 -> [w910]
              tunnel: w904 -> [w909]
              n134 = call <vilib>:"Butterworth Filter PtByPt.vi"("initialize"=w910, "order"=w909, "filter type"=Filter_Passband_Type."Lowpass", "low cutoff freq: fl"=w912, "sampling freq: fs"=w914, "x"=w915) -> ("Filtered x"=w913:dbl)  [unwired: 3 in, 1 out]
            }
          }
          frame 63 {
            n135 = for {
              tunnel: w916 -> [w929] mode=indexing
              tunnel: w921 -> [w926]
              tunnel: w922 -> [w928]
              tunnel: [w927] -> w917 mode=indexing
              tunnel: [w926] -> w920
              tunnel: w919 -> [w924]
              tunnel: w918 -> [w923]
              n136 = call <vilib>:"Butterworth Filter PtByPt.vi"("initialize"=w924, "order"=w923, "filter type"=Filter_Passband_Type."Lowpass", "low cutoff freq: fl"=w926, "sampling freq: fs"=w928, "x"=w929) -> ("Filtered x"=w927:dbl)  [unwired: 3 in, 1 out]
            }
          }
          frame 64 {
            n137 = for {
              tunnel: w930 -> [w943] mode=indexing
              tunnel: w935 -> [w940]
              tunnel: w936 -> [w942]
              tunnel: [w941] -> w931 mode=indexing
              tunnel: [w940] -> w934
              tunnel: w933 -> [w938]
              tunnel: w932 -> [w937]
              n138 = call <vilib>:"Butterworth Filter PtByPt.vi"("initialize"=w938, "order"=w937, "filter type"=Filter_Passband_Type."Lowpass", "low cutoff freq: fl"=w940, "sampling freq: fs"=w942, "x"=w943) -> ("Filtered x"=w941:dbl)  [unwired: 3 in, 1 out]
            }
          }
          frame 65 {
            n139 = for {
              tunnel: w944 -> [w957] mode=indexing
              tunnel: w949 -> [w954]
              tunnel: w950 -> [w956]
              tunnel: [w955] -> w945 mode=indexing
              tunnel: [w954] -> w948
              tunnel: w947 -> [w952]
              tunnel: w946 -> [w951]
              n140 = call <vilib>:"Butterworth Filter PtByPt.vi"("initialize"=w952, "order"=w951, "filter type"=Filter_Passband_Type."Lowpass", "low cutoff freq: fl"=w954, "sampling freq: fs"=w956, "x"=w957) -> ("Filtered x"=w955:dbl)  [unwired: 3 in, 1 out]
            }
          }
          frame 66 {
            n141 = for {
              tunnel: w958 -> [w971] mode=indexing
              tunnel: w963 -> [w968]
              tunnel: w964 -> [w970]
              tunnel: [w969] -> w959 mode=indexing
              tunnel: [w968] -> w962
              tunnel: w961 -> [w966]
              tunnel: w960 -> [w965]
              n142 = call <vilib>:"Butterworth Filter PtByPt.vi"("initialize"=w966, "order"=w965, "filter type"=Filter_Passband_Type."Lowpass", "low cutoff freq: fl"=w968, "sampling freq: fs"=w970, "x"=w971) -> ("Filtered x"=w969:dbl)  [unwired: 3 in, 1 out]
            }
          }
          frame 67 {
            n143 = for {
              tunnel: w972 -> [w985] mode=indexing
              tunnel: w977 -> [w982]
              tunnel: w978 -> [w984]
              tunnel: [w983] -> w973 mode=indexing
              tunnel: [w982] -> w976
              tunnel: w975 -> [w980]
              tunnel: w974 -> [w979]
              n144 = call <vilib>:"Butterworth Filter PtByPt.vi"("initialize"=w980, "order"=w979, "filter type"=Filter_Passband_Type."Lowpass", "low cutoff freq: fl"=w982, "sampling freq: fs"=w984, "x"=w985) -> ("Filtered x"=w983:dbl)  [unwired: 3 in, 1 out]
            }
          }
          frame 68 {
            n145 = for {
              tunnel: w986 -> [w999] mode=indexing
              tunnel: w991 -> [w996]
              tunnel: w992 -> [w998]
              tunnel: [w997] -> w987 mode=indexing
              tunnel: [w996] -> w990
              tunnel: w989 -> [w994]
              tunnel: w988 -> [w993]
              n146 = call <vilib>:"Butterworth Filter PtByPt.vi"("initialize"=w994, "order"=w993, "filter type"=Filter_Passband_Type."Lowpass", "low cutoff freq: fl"=w996, "sampling freq: fs"=w998, "x"=w999) -> ("Filtered x"=w997:dbl)  [unwired: 3 in, 1 out]
            }
          }
          frame 69 {
            n147 = for {
              tunnel: w1000 -> [w1013] mode=indexing
              tunnel: w1005 -> [w1010]
              tunnel: w1006 -> [w1012]
              tunnel: [w1011] -> w1001 mode=indexing
              tunnel: [w1010] -> w1004
              tunnel: w1003 -> [w1008]
              tunnel: w1002 -> [w1007]
              n148 = call <vilib>:"Butterworth Filter PtByPt.vi"("initialize"=w1008, "order"=w1007, "filter type"=Filter_Passband_Type."Lowpass", "low cutoff freq: fl"=w1010, "sampling freq: fs"=w1012, "x"=w1013) -> ("Filtered x"=w1011:dbl)  [unwired: 3 in, 1 out]
            }
          }
          frame 70 {
            n149 = for {
              tunnel: w1014 -> [w1027] mode=indexing
              tunnel: w1019 -> [w1024]
              tunnel: w1020 -> [w1026]
              tunnel: [w1025] -> w1015 mode=indexing
              tunnel: [w1024] -> w1018
              tunnel: w1017 -> [w1022]
              tunnel: w1016 -> [w1021]
              n150 = call <vilib>:"Butterworth Filter PtByPt.vi"("initialize"=w1022, "order"=w1021, "filter type"=Filter_Passband_Type."Lowpass", "low cutoff freq: fl"=w1024, "sampling freq: fs"=w1026, "x"=w1027) -> ("Filtered x"=w1025:dbl)  [unwired: 3 in, 1 out]
            }
          }
          frame 71 {
            n151 = for {
              tunnel: w1028 -> [w1041] mode=indexing
              tunnel: w1033 -> [w1038]
              tunnel: w1034 -> [w1040]
              tunnel: [w1039] -> w1029 mode=indexing
              tunnel: [w1038] -> w1032
              tunnel: w1031 -> [w1036]
              tunnel: w1030 -> [w1035]
              n152 = call <vilib>:"Butterworth Filter PtByPt.vi"("initialize"=w1036, "order"=w1035, "filter type"=Filter_Passband_Type."Lowpass", "low cutoff freq: fl"=w1038, "sampling freq: fs"=w1040, "x"=w1041) -> ("Filtered x"=w1039:dbl)  [unwired: 3 in, 1 out]
            }
          }
          frame 72 {
            n153 = for {
              tunnel: w1042 -> [w1055] mode=indexing
              tunnel: w1047 -> [w1052]
              tunnel: w1048 -> [w1054]
              tunnel: [w1053] -> w1043 mode=indexing
              tunnel: [w1052] -> w1046
              tunnel: w1045 -> [w1050]
              tunnel: w1044 -> [w1049]
              n154 = call <vilib>:"Butterworth Filter PtByPt.vi"("initialize"=w1050, "order"=w1049, "filter type"=Filter_Passband_Type."Lowpass", "low cutoff freq: fl"=w1052, "sampling freq: fs"=w1054, "x"=w1055) -> ("Filtered x"=w1053:dbl)  [unwired: 3 in, 1 out]
            }
          }
          frame 73 {
            n155 = for {
              tunnel: w1056 -> [w1069] mode=indexing
              tunnel: w1061 -> [w1066]
              tunnel: w1062 -> [w1068]
              tunnel: [w1067] -> w1057 mode=indexing
              tunnel: [w1066] -> w1060
              tunnel: w1059 -> [w1064]
              tunnel: w1058 -> [w1063]
              n156 = call <vilib>:"Butterworth Filter PtByPt.vi"("initialize"=w1064, "order"=w1063, "filter type"=Filter_Passband_Type."Lowpass", "low cutoff freq: fl"=w1066, "sampling freq: fs"=w1068, "x"=w1069) -> ("Filtered x"=w1067:dbl)  [unwired: 3 in, 1 out]
            }
          }
          frame 74 {
            n157 = for {
              tunnel: w1070 -> [w1083] mode=indexing
              tunnel: w1075 -> [w1080]
              tunnel: w1076 -> [w1082]
              tunnel: [w1081] -> w1071 mode=indexing
              tunnel: [w1080] -> w1074
              tunnel: w1073 -> [w1078]
              tunnel: w1072 -> [w1077]
              n158 = call <vilib>:"Butterworth Filter PtByPt.vi"("initialize"=w1078, "order"=w1077, "filter type"=Filter_Passband_Type."Lowpass", "low cutoff freq: fl"=w1080, "sampling freq: fs"=w1082, "x"=w1083) -> ("Filtered x"=w1081:dbl)  [unwired: 3 in, 1 out]
            }
          }
          frame 75 {
            n159 = for {
              tunnel: w1084 -> [w1097] mode=indexing
              tunnel: w1089 -> [w1094]
              tunnel: w1090 -> [w1096]
              tunnel: [w1095] -> w1085 mode=indexing
              tunnel: [w1094] -> w1088
              tunnel: w1087 -> [w1092]
              tunnel: w1086 -> [w1091]
              n160 = call <vilib>:"Butterworth Filter PtByPt.vi"("initialize"=w1092, "order"=w1091, "filter type"=Filter_Passband_Type."Lowpass", "low cutoff freq: fl"=w1094, "sampling freq: fs"=w1096, "x"=w1097) -> ("Filtered x"=w1095:dbl)  [unwired: 3 in, 1 out]
            }
          }
          frame 76 {
            n161 = for {
              tunnel: w1098 -> [w1111] mode=indexing
              tunnel: w1103 -> [w1108]
              tunnel: w1104 -> [w1110]
              tunnel: [w1109] -> w1099 mode=indexing
              tunnel: [w1108] -> w1102
              tunnel: w1101 -> [w1106]
              tunnel: w1100 -> [w1105]
              n162 = call <vilib>:"Butterworth Filter PtByPt.vi"("initialize"=w1106, "order"=w1105, "filter type"=Filter_Passband_Type."Lowpass", "low cutoff freq: fl"=w1108, "sampling freq: fs"=w1110, "x"=w1111) -> ("Filtered x"=w1109:dbl)  [unwired: 3 in, 1 out]
            }
          }
          frame 77 {
            n163 = for {
              tunnel: w1112 -> [w1125] mode=indexing
              tunnel: w1117 -> [w1122]
              tunnel: w1118 -> [w1124]
              tunnel: [w1123] -> w1113 mode=indexing
              tunnel: [w1122] -> w1116
              tunnel: w1115 -> [w1120]
              tunnel: w1114 -> [w1119]
              n164 = call <vilib>:"Butterworth Filter PtByPt.vi"("initialize"=w1120, "order"=w1119, "filter type"=Filter_Passband_Type."Lowpass", "low cutoff freq: fl"=w1122, "sampling freq: fs"=w1124, "x"=w1125) -> ("Filtered x"=w1123:dbl)  [unwired: 3 in, 1 out]
            }
          }
          frame 78 {
            n165 = for {
              tunnel: w1126 -> [w1139] mode=indexing
              tunnel: w1131 -> [w1136]
              tunnel: w1132 -> [w1138]
              tunnel: [w1137] -> w1127 mode=indexing
              tunnel: [w1136] -> w1130
              tunnel: w1129 -> [w1134]
              tunnel: w1128 -> [w1133]
              n166 = call <vilib>:"Butterworth Filter PtByPt.vi"("initialize"=w1134, "order"=w1133, "filter type"=Filter_Passband_Type."Lowpass", "low cutoff freq: fl"=w1136, "sampling freq: fs"=w1138, "x"=w1139) -> ("Filtered x"=w1137:dbl)  [unwired: 3 in, 1 out]
            }
          }
          frame 79 {
            n167 = for {
              tunnel: w1140 -> [w1153] mode=indexing
              tunnel: w1145 -> [w1150]
              tunnel: w1146 -> [w1152]
              tunnel: [w1151] -> w1141 mode=indexing
              tunnel: [w1150] -> w1144
              tunnel: w1143 -> [w1148]
              tunnel: w1142 -> [w1147]
              n168 = call <vilib>:"Butterworth Filter PtByPt.vi"("initialize"=w1148, "order"=w1147, "filter type"=Filter_Passband_Type."Lowpass", "low cutoff freq: fl"=w1150, "sampling freq: fs"=w1152, "x"=w1153) -> ("Filtered x"=w1151:dbl)  [unwired: 3 in, 1 out]
            }
          }
          frame 80 {
            n169 = for {
              tunnel: w1154 -> [w1167] mode=indexing
              tunnel: w1159 -> [w1164]
              tunnel: w1160 -> [w1166]
              tunnel: [w1165] -> w1155 mode=indexing
              tunnel: [w1164] -> w1158
              tunnel: w1157 -> [w1162]
              tunnel: w1156 -> [w1161]
              n170 = call <vilib>:"Butterworth Filter PtByPt.vi"("initialize"=w1162, "order"=w1161, "filter type"=Filter_Passband_Type."Lowpass", "low cutoff freq: fl"=w1164, "sampling freq: fs"=w1166, "x"=w1167) -> ("Filtered x"=w1165:dbl)  [unwired: 3 in, 1 out]
            }
          }
          frame 81 {
            n171 = for {
              tunnel: w1168 -> [w1181] mode=indexing
              tunnel: w1173 -> [w1178]
              tunnel: w1174 -> [w1180]
              tunnel: [w1179] -> w1169 mode=indexing
              tunnel: [w1178] -> w1172
              tunnel: w1171 -> [w1176]
              tunnel: w1170 -> [w1175]
              n172 = call <vilib>:"Butterworth Filter PtByPt.vi"("initialize"=w1176, "order"=w1175, "filter type"=Filter_Passband_Type."Lowpass", "low cutoff freq: fl"=w1178, "sampling freq: fs"=w1180, "x"=w1181) -> ("Filtered x"=w1179:dbl)  [unwired: 3 in, 1 out]
            }
          }
          frame 82 {
            n173 = for {
              tunnel: w1182 -> [w1195] mode=indexing
              tunnel: w1187 -> [w1192]
              tunnel: w1188 -> [w1194]
              tunnel: [w1193] -> w1183 mode=indexing
              tunnel: [w1192] -> w1186
              tunnel: w1185 -> [w1190]
              tunnel: w1184 -> [w1189]
              n174 = call <vilib>:"Butterworth Filter PtByPt.vi"("initialize"=w1190, "order"=w1189, "filter type"=Filter_Passband_Type."Lowpass", "low cutoff freq: fl"=w1192, "sampling freq: fs"=w1194, "x"=w1195) -> ("Filtered x"=w1193:dbl)  [unwired: 3 in, 1 out]
            }
          }
          frame 83 {
            n175 = for {
              tunnel: w1196 -> [w1209] mode=indexing
              tunnel: w1201 -> [w1206]
              tunnel: w1202 -> [w1208]
              tunnel: [w1207] -> w1197 mode=indexing
              tunnel: [w1206] -> w1200
              tunnel: w1199 -> [w1204]
              tunnel: w1198 -> [w1203]
              n176 = call <vilib>:"Butterworth Filter PtByPt.vi"("initialize"=w1204, "order"=w1203, "filter type"=Filter_Passband_Type."Lowpass", "low cutoff freq: fl"=w1206, "sampling freq: fs"=w1208, "x"=w1209) -> ("Filtered x"=w1207:dbl)  [unwired: 3 in, 1 out]
            }
          }
          frame 84 {
            n177 = for {
              tunnel: w1210 -> [w1223] mode=indexing
              tunnel: w1215 -> [w1220]
              tunnel: w1216 -> [w1222]
              tunnel: [w1221] -> w1211 mode=indexing
              tunnel: [w1220] -> w1214
              tunnel: w1213 -> [w1218]
              tunnel: w1212 -> [w1217]
              n178 = call <vilib>:"Butterworth Filter PtByPt.vi"("initialize"=w1218, "order"=w1217, "filter type"=Filter_Passband_Type."Lowpass", "low cutoff freq: fl"=w1220, "sampling freq: fs"=w1222, "x"=w1223) -> ("Filtered x"=w1221:dbl)  [unwired: 3 in, 1 out]
            }
          }
          frame 85 {
            n179 = for {
              tunnel: w1224 -> [w1237] mode=indexing
              tunnel: w1229 -> [w1234]
              tunnel: w1230 -> [w1236]
              tunnel: [w1235] -> w1225 mode=indexing
              tunnel: [w1234] -> w1228
              tunnel: w1227 -> [w1232]
              tunnel: w1226 -> [w1231]
              n180 = call <vilib>:"Butterworth Filter PtByPt.vi"("initialize"=w1232, "order"=w1231, "filter type"=Filter_Passband_Type."Lowpass", "low cutoff freq: fl"=w1234, "sampling freq: fs"=w1236, "x"=w1237) -> ("Filtered x"=w1235:dbl)  [unwired: 3 in, 1 out]
            }
          }
          frame 86 {
            n181 = for {
              tunnel: w1238 -> [w1251] mode=indexing
              tunnel: w1243 -> [w1248]
              tunnel: w1244 -> [w1250]
              tunnel: [w1249] -> w1239 mode=indexing
              tunnel: [w1248] -> w1242
              tunnel: w1241 -> [w1246]
              tunnel: w1240 -> [w1245]
              n182 = call <vilib>:"Butterworth Filter PtByPt.vi"("initialize"=w1246, "order"=w1245, "filter type"=Filter_Passband_Type."Lowpass", "low cutoff freq: fl"=w1248, "sampling freq: fs"=w1250, "x"=w1251) -> ("Filtered x"=w1249:dbl)  [unwired: 3 in, 1 out]
            }
          }
          frame 87 {
            n183 = for {
              tunnel: w1252 -> [w1265] mode=indexing
              tunnel: w1257 -> [w1262]
              tunnel: w1258 -> [w1264]
              tunnel: [w1263] -> w1253 mode=indexing
              tunnel: [w1262] -> w1256
              tunnel: w1255 -> [w1260]
              tunnel: w1254 -> [w1259]
              n184 = call <vilib>:"Butterworth Filter PtByPt.vi"("initialize"=w1260, "order"=w1259, "filter type"=Filter_Passband_Type."Lowpass", "low cutoff freq: fl"=w1262, "sampling freq: fs"=w1264, "x"=w1265) -> ("Filtered x"=w1263:dbl)  [unwired: 3 in, 1 out]
            }
          }
          frame 88 {
            n185 = for {
              tunnel: w1266 -> [w1279] mode=indexing
              tunnel: w1271 -> [w1276]
              tunnel: w1272 -> [w1278]
              tunnel: [w1277] -> w1267 mode=indexing
              tunnel: [w1276] -> w1270
              tunnel: w1269 -> [w1274]
              tunnel: w1268 -> [w1273]
              n186 = call <vilib>:"Butterworth Filter PtByPt.vi"("initialize"=w1274, "order"=w1273, "filter type"=Filter_Passband_Type."Lowpass", "low cutoff freq: fl"=w1276, "sampling freq: fs"=w1278, "x"=w1279) -> ("Filtered x"=w1277:dbl)  [unwired: 3 in, 1 out]
            }
          }
          frame 89 {
            n187 = for {
              tunnel: w1280 -> [w1293] mode=indexing
              tunnel: w1285 -> [w1290]
              tunnel: w1286 -> [w1292]
              tunnel: [w1291] -> w1281 mode=indexing
              tunnel: [w1290] -> w1284
              tunnel: w1283 -> [w1288]
              tunnel: w1282 -> [w1287]
              n188 = call <vilib>:"Butterworth Filter PtByPt.vi"("initialize"=w1288, "order"=w1287, "filter type"=Filter_Passband_Type."Lowpass", "low cutoff freq: fl"=w1290, "sampling freq: fs"=w1292, "x"=w1293) -> ("Filtered x"=w1291:dbl)  [unwired: 3 in, 1 out]
            }
          }
          frame 90 {
            n189 = for {
              tunnel: w1294 -> [w1307] mode=indexing
              tunnel: w1299 -> [w1304]
              tunnel: w1300 -> [w1306]
              tunnel: [w1305] -> w1295 mode=indexing
              tunnel: [w1304] -> w1298
              tunnel: w1297 -> [w1302]
              tunnel: w1296 -> [w1301]
              n190 = call <vilib>:"Butterworth Filter PtByPt.vi"("initialize"=w1302, "order"=w1301, "filter type"=Filter_Passband_Type."Lowpass", "low cutoff freq: fl"=w1304, "sampling freq: fs"=w1306, "x"=w1307) -> ("Filtered x"=w1305:dbl)  [unwired: 3 in, 1 out]
            }
          }
          frame 91 {
            n191 = for {
              tunnel: w1308 -> [w1321] mode=indexing
              tunnel: w1313 -> [w1318]
              tunnel: w1314 -> [w1320]
              tunnel: [w1319] -> w1309 mode=indexing
              tunnel: [w1318] -> w1312
              tunnel: w1311 -> [w1316]
              tunnel: w1310 -> [w1315]
              n192 = call <vilib>:"Butterworth Filter PtByPt.vi"("initialize"=w1316, "order"=w1315, "filter type"=Filter_Passband_Type."Lowpass", "low cutoff freq: fl"=w1318, "sampling freq: fs"=w1320, "x"=w1321) -> ("Filtered x"=w1319:dbl)  [unwired: 3 in, 1 out]
            }
          }
          frame 92 {
            n193 = for {
              tunnel: w1322 -> [w1335] mode=indexing
              tunnel: w1327 -> [w1332]
              tunnel: w1328 -> [w1334]
              tunnel: [w1333] -> w1323 mode=indexing
              tunnel: [w1332] -> w1326
              tunnel: w1325 -> [w1330]
              tunnel: w1324 -> [w1329]
              n194 = call <vilib>:"Butterworth Filter PtByPt.vi"("initialize"=w1330, "order"=w1329, "filter type"=Filter_Passband_Type."Lowpass", "low cutoff freq: fl"=w1332, "sampling freq: fs"=w1334, "x"=w1335) -> ("Filtered x"=w1333:dbl)  [unwired: 3 in, 1 out]
            }
          }
          frame 93 {
            n195 = for {
              tunnel: w1336 -> [w1349] mode=indexing
              tunnel: w1341 -> [w1346]
              tunnel: w1342 -> [w1348]
              tunnel: [w1347] -> w1337 mode=indexing
              tunnel: [w1346] -> w1340
              tunnel: w1339 -> [w1344]
              tunnel: w1338 -> [w1343]
              n196 = call <vilib>:"Butterworth Filter PtByPt.vi"("initialize"=w1344, "order"=w1343, "filter type"=Filter_Passband_Type."Lowpass", "low cutoff freq: fl"=w1346, "sampling freq: fs"=w1348, "x"=w1349) -> ("Filtered x"=w1347:dbl)  [unwired: 3 in, 1 out]
            }
          }
          frame 94 {
            n197 = for {
              tunnel: w1350 -> [w1363] mode=indexing
              tunnel: w1355 -> [w1360]
              tunnel: w1356 -> [w1362]
              tunnel: [w1361] -> w1351 mode=indexing
              tunnel: [w1360] -> w1354
              tunnel: w1353 -> [w1358]
              tunnel: w1352 -> [w1357]
              n198 = call <vilib>:"Butterworth Filter PtByPt.vi"("initialize"=w1358, "order"=w1357, "filter type"=Filter_Passband_Type."Lowpass", "low cutoff freq: fl"=w1360, "sampling freq: fs"=w1362, "x"=w1363) -> ("Filtered x"=w1361:dbl)  [unwired: 3 in, 1 out]
            }
          }
          frame 95 {
            n199 = for {
              tunnel: w1364 -> [w1377] mode=indexing
              tunnel: w1369 -> [w1374]
              tunnel: w1370 -> [w1376]
              tunnel: [w1375] -> w1365 mode=indexing
              tunnel: [w1374] -> w1368
              tunnel: w1367 -> [w1372]
              tunnel: w1366 -> [w1371]
              n200 = call <vilib>:"Butterworth Filter PtByPt.vi"("initialize"=w1372, "order"=w1371, "filter type"=Filter_Passband_Type."Lowpass", "low cutoff freq: fl"=w1374, "sampling freq: fs"=w1376, "x"=w1377) -> ("Filtered x"=w1375:dbl)  [unwired: 3 in, 1 out]
            }
          }
          frame 96 {
            n201 = for {
              tunnel: w1378 -> [w1391] mode=indexing
              tunnel: w1383 -> [w1388]
              tunnel: w1384 -> [w1390]
              tunnel: [w1389] -> w1379 mode=indexing
              tunnel: [w1388] -> w1382
              tunnel: w1381 -> [w1386]
              tunnel: w1380 -> [w1385]
              n202 = call <vilib>:"Butterworth Filter PtByPt.vi"("initialize"=w1386, "order"=w1385, "filter type"=Filter_Passband_Type."Lowpass", "low cutoff freq: fl"=w1388, "sampling freq: fs"=w1390, "x"=w1391) -> ("Filtered x"=w1389:dbl)  [unwired: 3 in, 1 out]
            }
          }
          frame 97 {
            n203 = for {
              tunnel: w1392 -> [w1405] mode=indexing
              tunnel: w1397 -> [w1402]
              tunnel: w1398 -> [w1404]
              tunnel: [w1403] -> w1393 mode=indexing
              tunnel: [w1402] -> w1396
              tunnel: w1395 -> [w1400]
              tunnel: w1394 -> [w1399]
              n204 = call <vilib>:"Butterworth Filter PtByPt.vi"("initialize"=w1400, "order"=w1399, "filter type"=Filter_Passband_Type."Lowpass", "low cutoff freq: fl"=w1402, "sampling freq: fs"=w1404, "x"=w1405) -> ("Filtered x"=w1403:dbl)  [unwired: 3 in, 1 out]
            }
          }
          frame 98 {
            n205 = for {
              tunnel: w1406 -> [w1419] mode=indexing
              tunnel: w1411 -> [w1416]
              tunnel: w1412 -> [w1418]
              tunnel: [w1417] -> w1407 mode=indexing
              tunnel: [w1416] -> w1410
              tunnel: w1409 -> [w1414]
              tunnel: w1408 -> [w1413]
              n206 = call <vilib>:"Butterworth Filter PtByPt.vi"("initialize"=w1414, "order"=w1413, "filter type"=Filter_Passband_Type."Lowpass", "low cutoff freq: fl"=w1416, "sampling freq: fs"=w1418, "x"=w1419) -> ("Filtered x"=w1417:dbl)  [unwired: 3 in, 1 out]
            }
          }
          frame 99 {
            n207 = for {
              tunnel: w1420 -> [w1433] mode=indexing
              tunnel: w1425 -> [w1430]
              tunnel: w1426 -> [w1432]
              tunnel: [w1431] -> w1421 mode=indexing
              tunnel: [w1430] -> w1424
              tunnel: w1423 -> [w1428]
              tunnel: w1422 -> [w1427]
              n208 = call <vilib>:"Butterworth Filter PtByPt.vi"("initialize"=w1428, "order"=w1427, "filter type"=Filter_Passband_Type."Lowpass", "low cutoff freq: fl"=w1430, "sampling freq: fs"=w1432, "x"=w1433) -> ("Filtered x"=w1431:dbl)  [unwired: 3 in, 1 out]
            }
          }
          frame 100 {
            n209 = for {
              tunnel: w1434 -> [w1447] mode=indexing
              tunnel: w1439 -> [w1444]
              tunnel: w1440 -> [w1446]
              tunnel: [w1445] -> w1435 mode=indexing
              tunnel: [w1444] -> w1438
              tunnel: w1437 -> [w1442]
              tunnel: w1436 -> [w1441]
              n210 = call <vilib>:"Butterworth Filter PtByPt.vi"("initialize"=w1442, "order"=w1441, "filter type"=Filter_Passband_Type."Lowpass", "low cutoff freq: fl"=w1444, "sampling freq: fs"=w1446, "x"=w1447) -> ("Filtered x"=w1445:dbl)  [unwired: 3 in, 1 out]
            }
          }
          frame 101 {
            n211 = for {
              tunnel: w1448 -> [w1461] mode=indexing
              tunnel: w1453 -> [w1458]
              tunnel: w1454 -> [w1460]
              tunnel: [w1459] -> w1449 mode=indexing
              tunnel: [w1458] -> w1452
              tunnel: w1451 -> [w1456]
              tunnel: w1450 -> [w1455]
              n212 = call <vilib>:"Butterworth Filter PtByPt.vi"("initialize"=w1456, "order"=w1455, "filter type"=Filter_Passband_Type."Lowpass", "low cutoff freq: fl"=w1458, "sampling freq: fs"=w1460, "x"=w1461) -> ("Filtered x"=w1459:dbl)  [unwired: 3 in, 1 out]
            }
          }
          frame 102 {
            n213 = for {
              tunnel: w1462 -> [w1475] mode=indexing
              tunnel: w1467 -> [w1472]
              tunnel: w1468 -> [w1474]
              tunnel: [w1473] -> w1463 mode=indexing
              tunnel: [w1472] -> w1466
              tunnel: w1465 -> [w1470]
              tunnel: w1464 -> [w1469]
              n214 = call <vilib>:"Butterworth Filter PtByPt.vi"("initialize"=w1470, "order"=w1469, "filter type"=Filter_Passband_Type."Lowpass", "low cutoff freq: fl"=w1472, "sampling freq: fs"=w1474, "x"=w1475) -> ("Filtered x"=w1473:dbl)  [unwired: 3 in, 1 out]
            }
          }
          frame 103 {
            n215 = for {
              tunnel: w1476 -> [w1489] mode=indexing
              tunnel: w1481 -> [w1486]
              tunnel: w1482 -> [w1488]
              tunnel: [w1487] -> w1477 mode=indexing
              tunnel: [w1486] -> w1480
              tunnel: w1479 -> [w1484]
              tunnel: w1478 -> [w1483]
              n216 = call <vilib>:"Butterworth Filter PtByPt.vi"("initialize"=w1484, "order"=w1483, "filter type"=Filter_Passband_Type."Lowpass", "low cutoff freq: fl"=w1486, "sampling freq: fs"=w1488, "x"=w1489) -> ("Filtered x"=w1487:dbl)  [unwired: 3 in, 1 out]
            }
          }
          frame 104 {
            n217 = for {
              tunnel: w1490 -> [w1503] mode=indexing
              tunnel: w1495 -> [w1500]
              tunnel: w1496 -> [w1502]
              tunnel: [w1501] -> w1491 mode=indexing
              tunnel: [w1500] -> w1494
              tunnel: w1493 -> [w1498]
              tunnel: w1492 -> [w1497]
              n218 = call <vilib>:"Butterworth Filter PtByPt.vi"("initialize"=w1498, "order"=w1497, "filter type"=Filter_Passband_Type."Lowpass", "low cutoff freq: fl"=w1500, "sampling freq: fs"=w1502, "x"=w1503) -> ("Filtered x"=w1501:dbl)  [unwired: 3 in, 1 out]
            }
          }
          frame 105 {
            n219 = for {
              tunnel: w1504 -> [w1517] mode=indexing
              tunnel: w1509 -> [w1514]
              tunnel: w1510 -> [w1516]
              tunnel: [w1515] -> w1505 mode=indexing
              tunnel: [w1514] -> w1508
              tunnel: w1507 -> [w1512]
              tunnel: w1506 -> [w1511]
              n220 = call <vilib>:"Butterworth Filter PtByPt.vi"("initialize"=w1512, "order"=w1511, "filter type"=Filter_Passband_Type."Lowpass", "low cutoff freq: fl"=w1514, "sampling freq: fs"=w1516, "x"=w1517) -> ("Filtered x"=w1515:dbl)  [unwired: 3 in, 1 out]
            }
          }
          frame 106 {
            n221 = for {
              tunnel: w1518 -> [w1531] mode=indexing
              tunnel: w1523 -> [w1528]
              tunnel: w1524 -> [w1530]
              tunnel: [w1529] -> w1519 mode=indexing
              tunnel: [w1528] -> w1522
              tunnel: w1521 -> [w1526]
              tunnel: w1520 -> [w1525]
              n222 = call <vilib>:"Butterworth Filter PtByPt.vi"("initialize"=w1526, "order"=w1525, "filter type"=Filter_Passband_Type."Lowpass", "low cutoff freq: fl"=w1528, "sampling freq: fs"=w1530, "x"=w1531) -> ("Filtered x"=w1529:dbl)  [unwired: 3 in, 1 out]
            }
          }
          frame 107 {
            n223 = for {
              tunnel: w1532 -> [w1545] mode=indexing
              tunnel: w1537 -> [w1542]
              tunnel: w1538 -> [w1544]
              tunnel: [w1543] -> w1533 mode=indexing
              tunnel: [w1542] -> w1536
              tunnel: w1535 -> [w1540]
              tunnel: w1534 -> [w1539]
              n224 = call <vilib>:"Butterworth Filter PtByPt.vi"("initialize"=w1540, "order"=w1539, "filter type"=Filter_Passband_Type."Lowpass", "low cutoff freq: fl"=w1542, "sampling freq: fs"=w1544, "x"=w1545) -> ("Filtered x"=w1543:dbl)  [unwired: 3 in, 1 out]
            }
          }
          frame 108 {
            n225 = for {
              tunnel: w1546 -> [w1559] mode=indexing
              tunnel: w1551 -> [w1556]
              tunnel: w1552 -> [w1558]
              tunnel: [w1557] -> w1547 mode=indexing
              tunnel: [w1556] -> w1550
              tunnel: w1549 -> [w1554]
              tunnel: w1548 -> [w1553]
              n226 = call <vilib>:"Butterworth Filter PtByPt.vi"("initialize"=w1554, "order"=w1553, "filter type"=Filter_Passband_Type."Lowpass", "low cutoff freq: fl"=w1556, "sampling freq: fs"=w1558, "x"=w1559) -> ("Filtered x"=w1557:dbl)  [unwired: 3 in, 1 out]
            }
          }
          frame 109 {
            n227 = for {
              tunnel: w1560 -> [w1573] mode=indexing
              tunnel: w1565 -> [w1570]
              tunnel: w1566 -> [w1572]
              tunnel: [w1571] -> w1561 mode=indexing
              tunnel: [w1570] -> w1564
              tunnel: w1563 -> [w1568]
              tunnel: w1562 -> [w1567]
              n228 = call <vilib>:"Butterworth Filter PtByPt.vi"("initialize"=w1568, "order"=w1567, "filter type"=Filter_Passband_Type."Lowpass", "low cutoff freq: fl"=w1570, "sampling freq: fs"=w1572, "x"=w1573) -> ("Filtered x"=w1571:dbl)  [unwired: 3 in, 1 out]
            }
          }
          frame 110 {
            n229 = for {
              tunnel: w1574 -> [w1587] mode=indexing
              tunnel: w1579 -> [w1584]
              tunnel: w1580 -> [w1586]
              tunnel: [w1585] -> w1575 mode=indexing
              tunnel: [w1584] -> w1578
              tunnel: w1577 -> [w1582]
              tunnel: w1576 -> [w1581]
              n230 = call <vilib>:"Butterworth Filter PtByPt.vi"("initialize"=w1582, "order"=w1581, "filter type"=Filter_Passband_Type."Lowpass", "low cutoff freq: fl"=w1584, "sampling freq: fs"=w1586, "x"=w1587) -> ("Filtered x"=w1585:dbl)  [unwired: 3 in, 1 out]
            }
          }
          frame 111 {
            n231 = for {
              tunnel: w1588 -> [w1601] mode=indexing
              tunnel: w1593 -> [w1598]
              tunnel: w1594 -> [w1600]
              tunnel: [w1599] -> w1589 mode=indexing
              tunnel: [w1598] -> w1592
              tunnel: w1591 -> [w1596]
              tunnel: w1590 -> [w1595]
              n232 = call <vilib>:"Butterworth Filter PtByPt.vi"("initialize"=w1596, "order"=w1595, "filter type"=Filter_Passband_Type."Lowpass", "low cutoff freq: fl"=w1598, "sampling freq: fs"=w1600, "x"=w1601) -> ("Filtered x"=w1599:dbl)  [unwired: 3 in, 1 out]
            }
          }
          frame 112 {
            n233 = for {
              tunnel: w1602 -> [w1615] mode=indexing
              tunnel: w1607 -> [w1612]
              tunnel: w1608 -> [w1614]
              tunnel: [w1613] -> w1603 mode=indexing
              tunnel: [w1612] -> w1606
              tunnel: w1605 -> [w1610]
              tunnel: w1604 -> [w1609]
              n234 = call <vilib>:"Butterworth Filter PtByPt.vi"("initialize"=w1610, "order"=w1609, "filter type"=Filter_Passband_Type."Lowpass", "low cutoff freq: fl"=w1612, "sampling freq: fs"=w1614, "x"=w1615) -> ("Filtered x"=w1613:dbl)  [unwired: 3 in, 1 out]
            }
          }
          frame 113 {
            n235 = for {
              tunnel: w1616 -> [w1629] mode=indexing
              tunnel: w1621 -> [w1626]
              tunnel: w1622 -> [w1628]
              tunnel: [w1627] -> w1617 mode=indexing
              tunnel: [w1626] -> w1620
              tunnel: w1619 -> [w1624]
              tunnel: w1618 -> [w1623]
              n236 = call <vilib>:"Butterworth Filter PtByPt.vi"("initialize"=w1624, "order"=w1623, "filter type"=Filter_Passband_Type."Lowpass", "low cutoff freq: fl"=w1626, "sampling freq: fs"=w1628, "x"=w1629) -> ("Filtered x"=w1627:dbl)  [unwired: 3 in, 1 out]
            }
          }
          frame 114 {
            n237 = for {
              tunnel: w1630 -> [w1643] mode=indexing
              tunnel: w1635 -> [w1640]
              tunnel: w1636 -> [w1642]
              tunnel: [w1641] -> w1631 mode=indexing
              tunnel: [w1640] -> w1634
              tunnel: w1633 -> [w1638]
              tunnel: w1632 -> [w1637]
              n238 = call <vilib>:"Butterworth Filter PtByPt.vi"("initialize"=w1638, "order"=w1637, "filter type"=Filter_Passband_Type."Lowpass", "low cutoff freq: fl"=w1640, "sampling freq: fs"=w1642, "x"=w1643) -> ("Filtered x"=w1641:dbl)  [unwired: 3 in, 1 out]
            }
          }
          frame 115 {
            n239 = for {
              tunnel: w1644 -> [w1657] mode=indexing
              tunnel: w1649 -> [w1654]
              tunnel: w1650 -> [w1656]
              tunnel: [w1655] -> w1645 mode=indexing
              tunnel: [w1654] -> w1648
              tunnel: w1647 -> [w1652]
              tunnel: w1646 -> [w1651]
              n240 = call <vilib>:"Butterworth Filter PtByPt.vi"("initialize"=w1652, "order"=w1651, "filter type"=Filter_Passband_Type."Lowpass", "low cutoff freq: fl"=w1654, "sampling freq: fs"=w1656, "x"=w1657) -> ("Filtered x"=w1655:dbl)  [unwired: 3 in, 1 out]
            }
          }
          frame 116 {
            n241 = for {
              tunnel: w1658 -> [w1671] mode=indexing
              tunnel: w1663 -> [w1668]
              tunnel: w1664 -> [w1670]
              tunnel: [w1669] -> w1659 mode=indexing
              tunnel: [w1668] -> w1662
              tunnel: w1661 -> [w1666]
              tunnel: w1660 -> [w1665]
              n242 = call <vilib>:"Butterworth Filter PtByPt.vi"("initialize"=w1666, "order"=w1665, "filter type"=Filter_Passband_Type."Lowpass", "low cutoff freq: fl"=w1668, "sampling freq: fs"=w1670, "x"=w1671) -> ("Filtered x"=w1669:dbl)  [unwired: 3 in, 1 out]
            }
          }
          frame 117 {
            n243 = for {
              tunnel: w1672 -> [w1685] mode=indexing
              tunnel: w1677 -> [w1682]
              tunnel: w1678 -> [w1684]
              tunnel: [w1683] -> w1673 mode=indexing
              tunnel: [w1682] -> w1676
              tunnel: w1675 -> [w1680]
              tunnel: w1674 -> [w1679]
              n244 = call <vilib>:"Butterworth Filter PtByPt.vi"("initialize"=w1680, "order"=w1679, "filter type"=Filter_Passband_Type."Lowpass", "low cutoff freq: fl"=w1682, "sampling freq: fs"=w1684, "x"=w1685) -> ("Filtered x"=w1683:dbl)  [unwired: 3 in, 1 out]
            }
          }
          frame 118 {
            n245 = for {
              tunnel: w1686 -> [w1699] mode=indexing
              tunnel: w1691 -> [w1696]
              tunnel: w1692 -> [w1698]
              tunnel: [w1697] -> w1687 mode=indexing
              tunnel: [w1696] -> w1690
              tunnel: w1689 -> [w1694]
              tunnel: w1688 -> [w1693]
              n246 = call <vilib>:"Butterworth Filter PtByPt.vi"("initialize"=w1694, "order"=w1693, "filter type"=Filter_Passband_Type."Lowpass", "low cutoff freq: fl"=w1696, "sampling freq: fs"=w1698, "x"=w1699) -> ("Filtered x"=w1697:dbl)  [unwired: 3 in, 1 out]
            }
          }
          frame 119 {
            n247 = for {
              tunnel: w1700 -> [w1713] mode=indexing
              tunnel: w1705 -> [w1710]
              tunnel: w1706 -> [w1712]
              tunnel: [w1711] -> w1701 mode=indexing
              tunnel: [w1710] -> w1704
              tunnel: w1703 -> [w1708]
              tunnel: w1702 -> [w1707]
              n248 = call <vilib>:"Butterworth Filter PtByPt.vi"("initialize"=w1708, "order"=w1707, "filter type"=Filter_Passband_Type."Lowpass", "low cutoff freq: fl"=w1710, "sampling freq: fs"=w1712, "x"=w1713) -> ("Filtered x"=w1711:dbl)  [unwired: 3 in, 1 out]
            }
          }
          frame 120 {
            n249 = for {
              tunnel: w1714 -> [w1727] mode=indexing
              tunnel: w1719 -> [w1724]
              tunnel: w1720 -> [w1726]
              tunnel: [w1725] -> w1715 mode=indexing
              tunnel: [w1724] -> w1718
              tunnel: w1717 -> [w1722]
              tunnel: w1716 -> [w1721]
              n250 = call <vilib>:"Butterworth Filter PtByPt.vi"("initialize"=w1722, "order"=w1721, "filter type"=Filter_Passband_Type."Lowpass", "low cutoff freq: fl"=w1724, "sampling freq: fs"=w1726, "x"=w1727) -> ("Filtered x"=w1725:dbl)  [unwired: 3 in, 1 out]
            }
          }
          frame 121 {
            n251 = for {
              tunnel: w1728 -> [w1741] mode=indexing
              tunnel: w1733 -> [w1738]
              tunnel: w1734 -> [w1740]
              tunnel: [w1739] -> w1729 mode=indexing
              tunnel: [w1738] -> w1732
              tunnel: w1731 -> [w1736]
              tunnel: w1730 -> [w1735]
              n252 = call <vilib>:"Butterworth Filter PtByPt.vi"("initialize"=w1736, "order"=w1735, "filter type"=Filter_Passband_Type."Lowpass", "low cutoff freq: fl"=w1738, "sampling freq: fs"=w1740, "x"=w1741) -> ("Filtered x"=w1739:dbl)  [unwired: 3 in, 1 out]
            }
          }
          frame 122 {
            n253 = for {
              tunnel: w1742 -> [w1755] mode=indexing
              tunnel: w1747 -> [w1752]
              tunnel: w1748 -> [w1754]
              tunnel: [w1753] -> w1743 mode=indexing
              tunnel: [w1752] -> w1746
              tunnel: w1745 -> [w1750]
              tunnel: w1744 -> [w1749]
              n254 = call <vilib>:"Butterworth Filter PtByPt.vi"("initialize"=w1750, "order"=w1749, "filter type"=Filter_Passband_Type."Lowpass", "low cutoff freq: fl"=w1752, "sampling freq: fs"=w1754, "x"=w1755) -> ("Filtered x"=w1753:dbl)  [unwired: 3 in, 1 out]
            }
          }
          frame 123 {
            n255 = for {
              tunnel: w1756 -> [w1769] mode=indexing
              tunnel: w1761 -> [w1766]
              tunnel: w1762 -> [w1768]
              tunnel: [w1767] -> w1757 mode=indexing
              tunnel: [w1766] -> w1760
              tunnel: w1759 -> [w1764]
              tunnel: w1758 -> [w1763]
              n256 = call <vilib>:"Butterworth Filter PtByPt.vi"("initialize"=w1764, "order"=w1763, "filter type"=Filter_Passband_Type."Lowpass", "low cutoff freq: fl"=w1766, "sampling freq: fs"=w1768, "x"=w1769) -> ("Filtered x"=w1767:dbl)  [unwired: 3 in, 1 out]
            }
          }
        }
        n257 = Bundle By Name(cluster=w25, "Y"=w28) -> (w24:waveform(dbl))
        n258 = in-place-array #1(w24) -> (w16:waveform(dbl)[])  [unwired: 1 out]
      }
    }
  }
  "Array out" <- w4
